vi "SCMP - Main Program v4.vi"() -> ()   [LabVIEW 2014]
doc: "Goodrich Exposure Range: .05microseconds to 798.9ms\n\nLow Gain (110e-/ADU)\nHigh Gain (6.5 e-/ADU)\n\nGA1280J Trigger Modes\n0 : Internally triggered; Internally timed\n1 : Externally triggered; Internally timed\n2 : Externally triggered; Externally timed\n3 : Externally gated; Internally timed\n\nFor list of camera commands\nsee Appendix A in the manual\n\n\nUse this template to build a standard state machine design pattern. Each state executes code and determines which state to transition to. Contrast this design pattern with the User Interface Event Handler pattern, in which code executes in response to user actions. Contrast this design pattern also with the Queued Message Handler pattern, in which each message handling code can queue zero or more new messages.\nNote: This template does not contain the most recent programming guidelines recommended by National Instruments. For a complete, project-based implementation of the Standard State Machine pattern, use the Create Project dialog box instead of this template."
uses:
  AISAS/Controls/Diffuser.ctl
  AISAS/Controls/Rotation.ctl
  PI/PI Control.ctl
  Controls/SCD - EDT - Emission Line Filter Wheel.ctl
  Controls/SCD - FITS Cluster.ctl
  AISAS/Mech/AISAS Mech.lvclass
  Controls/FITS Data type.ctl
  Controls/SCD - Calibration Optics Filter Wheel.ctl
  Controls/CoMP-S Controls/Polarization Optics Filter Wheel.ctl
  Controls/CoMP-S Controls/Emission Line Filter Wheel.ctl
  AISAS/Controls/focus.ctl
  Controls/peripherals.ctl
  Controls/Cameras select.ctl
  Controls/beaning.ctl
  Controls/Cookbook.ctl
  Controls/Cbk Data type.ctl
  Controls/Main Program States.ctl
  AISAS/Controls/motor.ctl
  AISAS/Mech/AISAS Mech.lvclass/AISAS Mech.ctl
  Camera/Andor Neo/Andor.lvclass
  Camera/Camera/Camera.lvclass
  Globals/Global - All Loop Stop.vi
  Globals/Global - pR netw comm.vi
  Controls/Globals.vi
  Controls/Global demo.vi
  c:/Users/mhutar/Documents/miro_lvproj/SCMP/Ancillary/Watlow EZ-ZONE/Public/Watbus.dll
  Ancillary/Watlow EZ-ZONE/Public/Watbus.dll
  <vilib>/Utility/error.llb/DialogType.ctl
panel:
  in  "Print scr1":bool
  in  "Comment":string="CoMP-S obs_prog_XXX"
  in  "Observer":string="Surname of the observer"
  out "Instrument":string
  out "Main Loop":bool
  out "Log Loop":bool
  out "Program":bool
  out "Version":string
  in  "AOI Width 2":i64=2560
  in  "AOI Height 2":i64=2160
  out "Latest Actions":string="\r"
  out "cbk name":string="automated_find_focus_656.cbk"
  out "Main Loop Error":errorcluster={"status"=TRUE, "code"=0, "source"=""}
  in  "Tab Control":T1(tab)
  in  "Auto scale":bool=TRUE
  in  "Live Preview":bool
  in  "Snap Images":bool
  out "Camera T Image Zoom":u16[][](graph)
  out "Histogram Graph 2":T2(graph)
  out "Timestamp 2":timestamp=timestamp(3507746192.5616717 s since 1904-01-01)
  out "Mean ADU 2":dbl=7788.0 format="%.1f"
  out "Sharpness 2":dbl format="%.2f"
  out "Camera FITS file path 2":path
  out "Camera R Image":u16[][](graph)
  in  "PI cam3 (mm)":T3 min=0.1 max=21.0 step=0.1 format="%.1f"
  in  "PI cam2 (mm)":T3 min=0.1 max=27.0 step=0.1 format="%.1f"
  in  "Calibration Optics":T4
  in  "Size":dbl format="%.2f"
  in  "Focus":T5 min=70.0 max=152.0 format="%.2f"
  in  "Andover Filter Wheel":T6
  in  "Calibration Wheel":T7
  in  "Binning":T8
  in  "Save Data to FITS?":bool
  out "Histogram Graph":T2(graph)
  in  "Exposure (s)":dbl=0.02 min=1e-05 max=10.0 step=0.001 format="%_3p"
  out "Timestamp":timestamp=timestamp(3507746192.5616717 s since 1904-01-01)
  in  "PI cam1 (mm)":T3 min=0.1 max=27.0 step=0.1 format="%.1f"
  out "Camera FITS file path":path
  in  "Emission Line Filters":T9
  in  "Set Filter Wheels":bool
  out "Mean ADU":dbl=7788.0 format="%.1f"
  out "Sharpness":dbl format="%.2f"
  in  "Diffuser":T10=enum."In Beam"
  in  "Rotation [deg]":T11 min=0.0 max=360.0 step=1.0 format="%.1f"
  in  "Move AISAS Mechanisms":bool
  in  "Motors":bool=TRUE
  out "Camera Image":u32[][](graph)
  out "Camera T Image":u16[][](graph)
  in  "Wavelength [nm]":dbl=557.0 min=0.0 step=0.01 format="%.2f"
  in  "Cameras":T12
  in  "preset cbk":u16(ring) caption="focus/filter/PIs/texp" items=["530.3nm (Fe XIV)", "587.6nm (He I D3)", "637.5nm (Fe X)", "656.3nm (H-Alpha)", "854.2nm (Ca I)", "1074.7nm (Fe XIII)", "1079.8nm (Fe XIII)", "1083.0nm (He I)"]
  in  "Setup Cor":bool
  in  "Looback disable":bool=TRUE caption="Disable Pointer Loopback\n  during Data aquisition"
  out "max Cookbook FPS":dbl=200.0 format="%#_3p"
  in  "Run Cookbook":bool
  in  "Save Data to FITS?":bool=TRUE
  out "Cookbook":T13=[{"Data Type"=enum."ACQUIRE DATA", "Arg 1"=0.0, "Arg 2"=0.0, "Arg 3"=path "", "Comments"=""}, {"Data Type"=enum."ACQUIRE DATA", "Arg 1"=0.0, "Arg 2"=0.0, "Arg 3"=path "", "Comments"=""}]
  out "FITS Path from Last Recipe Acquiring Data":path
  out "# of Recipes":i16
  out "Selected Cookbook":path
  out "Recipe Files":string[](array[string])
  in  "limit max Cookbook FPS to:":dbl=49.0 min=0.01 max=49.0 step=1.0 format="%_2f"
  out "Continually Read Log File":string="20160903-07:42:55 Live Preview Images\n20160903-07:44:38 Program Terminated\n20160903-07:45:16 Program Started\n20160903-07:45:18 Snap Single Image\n20160903-07:45:27 Live Preview Images\n20160903-07:46:17 Calibration & Filter wheel position:\t8\t5\n20160903-07:46:35 Live Preview Images\n20160903-07:50:39 Live Preview Images\n20160903-07:51:54 Camera Moved to Positon:-18.00\n20160903-07:51:55 Snap Single Image\n20160903-07:52:37 Loaded Cookbook\tfind_focus_656.cbk\n20160903-07:53:52 Run Cookbook\tfind_focus_656.cbk\n20160903-07:53:52 Recipe#0-exposure-20ms.rcp\n20160903-07:53:52 Recipe#1-fw-656.rcp\n20160903-07:53:54 Recipe#2-cal-open.rcp\n20160903-07:53:56 Recipe#3-move-absolute-neg19.rcp\n20160903-07:53:56 Recipe#4-take_656_focus_image.rcp\n20160903-07:54:02 Recipe#5-move-relative-neg0pt25.rcp\n20160903-07:55:56 Program Started\n20160903-07:56:02 Camera Moved to Positon:-18.00\n20160903-07:56:03 Snap Single Image\n20160903-07:56:35 Camera Moved to Positon:-19.00\n20160903-07:56:37 Snap Single Image\n20160903-07:56:58 Camera Moved to Positon:-20.00\n20160903-07:57:02 Snap Single Image\n20160903-07:57:20 Camera Moved to Positon:-21.00\n20160903-07:57:23 Snap Single Image\n20160903-07:57:36 Camera Moved to Positon:-22.00\n20160903-07:57:37 Snap Single Image\n20160903-07:57:53 Camera Moved to Positon:-25.00\n20160903-07:57:57 Snap Single Image\n20160903-07:58:13 Camera Moved to Positon:-30.00\n20160903-07:58:17 Snap Single Image\n20160903-07:58:43 Camera Moved to Positon:-18.00\n20160903-07:58:44 Snap Single Image\n20160903-07:58:58 Camera Moved to Positon:-17.00\n20160903-07:59:00 Snap Single Image\n20160903-08:00:39 Calibration & Filter wheel position:\t7\t6\n20160903-08:00:48 Snap Single Image\n20160903-08:01:42 Camera Moved to Positon:-65.00\n20160903-08:01:47 Snap Single Image\n20160903-08:02:07 Camera Moved to Positon:-70.00\n20160903-08:02:10 Snap Single Image\n20160903-08:02:51 Camera Moved to Positon:-75.00\n20160903-08:02:53 Snap Single Image\n20160903-08:03:25 Calibration & Filter wheel position:\t7\t7\n20160903-08:03:37 Snap Single Image\n20160903-08:03:55 Camera Moved to Positon:-76.00\n20160903-08:04:01 Snap Single Image\n20160903-08:04:13 Camera Moved to Positon:-77.00\n20160903-08:04:14 Snap Single Image\n20160903-08:04:24 Camera Moved to Positon:-78.00\n20160903-08:04:26 Snap Single Image\n20160903-08:04:38 Camera Moved to Positon:-79.00\n20160903-08:04:39 Snap Single Image\n20160903-08:04:50 Camera Moved to Positon:-83.00\n20160903-08:04:52 Snap Single Image\n20160903-08:05:10 Camera Moved to Positon:-73.00\n20160903-08:05:11 Snap Single Image\n20160903-08:05:22 Camera Moved to Positon:-71.00\n20160903-08:05:24 Snap Single Image\n20160903-08:05:34 Camera Moved to Positon:-69.00\n20160903-08:05:35 Snap Single Image\n20160903-08:05:47 Camera Moved to Positon:-67.00\n20160903-08:05:48 Snap Single Image\n20160903-08:06:13 Calibration & Filter wheel position:\t7\t8\n20160903-08:07:06 Snap Single Image\n20160903-08:07:17 Camera Moved to Positon:-69.00\n20160903-08:07:18 Snap Single Image\n20160903-08:07:28 Camera Moved to Positon:-71.00\n20160903-08:07:30 Snap Single Image\n20160903-08:07:40 Camera Moved to Positon:-73.00\n20160903-08:07:43 Snap Single Image\n20160903-08:07:53 Camera Moved to Positon:-75.00\n20160903-08:07:55 Snap Single Image\n20160903-08:08:04 Camera Moved to Positon:-77.00\n20160903-08:08:06 Snap Single Image\n20160903-08:08:17 Camera Moved to Positon:-79.00\n20160903-08:08:28 Snap Single Image\n20160903-08:08:43 Camera Moved to Positon:-81.00\n20160903-08:08:46 Snap Single Image\n20160903-08:09:05 Calibration & Filter wheel position:\t7\t9\n20160903-08:09:48 Camera Moved to Positon:-100.00\n20160903-08:09:50 Snap Single Image\n20160903-08:10:09 Snap Single Image\n20160903-08:10:26 Camera Moved to Positon:-100.00\n20160903-08:10:35 Camera Moved to Positon:-100.00\n20160903-08:10:37 Snap Single Image\n20160903-08:10:54 Camera Moved to Positon:-100.00\n20160903-08:10:59 Program Terminated\n20160903-08:12:25 Program Started\n20160903-08:12:33 Camera Moved to Positon:-100.00\n20160903-08:12:38 Program Terminated\n20160903-08:13:25 Program Started\n20160903-08:13:30 Camera Moved to Positon:-100.00\n20160903-08:13:37 Program Terminated\n20160903-08:14:12 Program Started\n20160903-08:14:19 Camera Moved to Positon:-100.00\n20160903-08:14:22 Snap Single Image\n20160903-08:14:37 Calibration & Filter wheel position:\t7\t9\n20160903-08:14:45 Snap Single Image\n20160903-08:14:56 Camera Moved to Positon:-105.00\n20160903-08:14:57 Snap Single Image\n20160903-08:15:10 Camera Moved to Positon:-110.00\n20160903-08:15:11 Snap Single Image\n20160903-08:15:23 Camera Moved to Positon:-115.00\n20160903-08:15:27 Snap Single Image\n20160903-08:15:39 Camera Moved to Positon:-120.00\n20160903-08:15:40 Snap Single Image\n20160903-08:15:59 Snap Single Image\n20160903-08:16:10 Camera Moved to Positon:-115.00\n20160903-08:16:11 Snap Single Image\n20160903-08:16:21 Camera Moved to Positon:-110.00\n20160903-08:16:22 Snap Single Image\n20160903-08:16:33 Camera Moved to Positon:-105.00\n20160903-08:16:36 Snap Single Image\n20160903-08:16:49 Camera Moved to Positon:-100.00\n20160903-08:16:51 Snap Single Image\n20160903-08:17:03 Camera Moved to Positon:-95.00\n20160903-08:17:05 Snap Single Image\n20160903-08:17:16 Camera Moved to Positon:-90.00\n20160903-08:17:18 Snap Single Image\n20160903-08:17:46 Camera Moved to Positon:-85.00\n20160903-08:17:49 Snap Single Image\n20160903-08:18:00 Camera Moved to Positon:-80.00\n20160903-08:18:02 Snap Single Image\n20160903-08:18:40 Calibration & Filter wheel position:\t7\t4\n20160903-08:18:59 Camera Moved to Positon:-20.00\n20160903-08:19:11 Snap Single Image\n20160903-08:19:23 Camera Moved to Positon:-18.00\n20160903-08:19:25 Snap Single Image\n20160903-08:19:38 Camera Moved to Positon:-22.00\n20160903-08:19:39 Snap Single Image\n20160903-08:19:51 Camera Moved to Positon:-24.00\n20160903-08:19:52 Snap Single Image\n20160903-08:20:04 Calibration & Filter wheel position:\t7\t3\n20160903-08:20:11 Snap Single Image\n20160903-08:20:22 Camera Moved to Positon:-18.00\n20160903-08:20:24 Snap Single Image\n20160903-08:20:39 Camera Moved to Positon:-16.00\n20160903-08:20:40 Snap Single Image\n20160903-08:20:53 Camera Moved to Positon:-14.00\n20160903-08:20:56 Snap Single Image\n20160903-08:21:06 Camera Moved to Positon:-12.00\n20160903-08:21:07 Snap Single Image\n20160903-08:21:16 Camera Moved to Positon:-10.00\n20160903-08:21:24 Snap Single Image\n20160903-08:21:34 Camera Moved to Positon: -8.00\n20160903-08:21:36 Snap Single Image\n20160903-08:22:12 Camera Moved to Positon: -6.00\n20160903-08:22:21 Snap Single Image\n20160903-08:23:09 Calibration & Filter wheel position:\t7\t1\n20160903-08:23:17 Snap Single Image\n20160903-08:23:27 Camera Moved to Positon: -4.00\n20160903-08:23:29 Snap Single Image\n20160903-08:23:37 Camera Moved to Positon: -2.00\n20160903-08:23:38 Snap Single Image\n20160903-08:23:47 Camera Moved to Positon:  0.00\n20160903-08:23:50 Snap Single Image\n20160903-08:26:00 Camera Moved to Positon:-18.00\n20160903-08:26:44 Program Started\n20160903-08:26:59 Camera Moved to Positon:-18.00\n20160903-08:27:05 Loaded Cookbook\tfind_focus_656.cbk\n20160903-08:27:12 Run Cookbook\tfind_focus_656.cbk\n20160903-08:27:12 Recipe#0-exposure-20ms.rcp\n20160903-08:27:12 Recipe#1-fw-656.rcp\n20160903-08:27:14 Recipe#2-cal-open.rcp\n20160903-08:27:16 Recipe#3-take_656_focus_image.rcp\n20160903-08:29:11 Camera Moved to Positon:-19.00\n20160903-08:29:17 Run Cookbook\tfind_focus_656.cbk\n20160903-08:29:17 Recipe#0-exposure-20ms.rcp\n20160903-08:29:17 Recipe#1-fw-656.rcp\n20160903-08:29:19 Recipe#2-cal-open.rcp\n20160903-08:29:21 Recipe#3-take_656_focus_image.rcp\n20160903-08:29:59 Camera Moved to Positon:-20.00\n20160903-08:30:03 Run Cookbook\tfind_focus_656.cbk\n20160903-08:30:03 Recipe#0-exposure-20ms.rcp\n20160903-08:30:03 Recipe#1-fw-656.rcp\n20160903-08:30:05 Recipe#2-cal-open.rcp\n20160903-08:30:07 Recipe#3-take_656_focus_image.rcp\n20160903-08:30:28 Camera Moved to Positon:-21.00\n20160903-08:30:32 Run Cookbook\tfind_focus_656.cbk\n20160903-08:30:32 Recipe#0-exposure-20ms.rcp\n20160903-08:30:32 Recipe#1-fw-656.rcp\n20160903-08:30:34 Recipe#2-cal-open.rcp\n20160903-08:30:36 Recipe#3-take_656_focus_image.rcp\n20160903-08:31:03 Camera Moved to Positon:-22.00\n20160903-08:31:06 Run Cookbook\tfind_focus_656.cbk\n20160903-08:31:06 Recipe#0-exposure-20ms.rcp\n20160903-08:31:06 Recipe#1-fw-656.rcp\n20160903-08:31:08 Recipe#2-cal-open.rcp\n20160903-08:31:10 Recipe#3-take_656_focus_image.rcp\n20160903-08:31:33 Camera Moved to Positon:-23.00\n20160903-08:31:38 Run Cookbook\tfind_focus_656.cbk\n20160903-08:31:38 Recipe#0-exposure-20ms.rcp\n20160903-08:31:38 Recipe#1-fw-656.rcp\n20160903-08:31:40 Recipe#2-cal-open.rcp\n20160903-08:31:42 Recipe#3-take_656_focus_image.rcp\n20160903-08:32:05 Camera Moved to Positon:-24.00\n20160903-08:32:08 Run Cookbook\tfind_focus_656.cbk\n20160903-08:32:08 Recipe#0-exposure-20ms.rcp\n20160903-08:32:08 Recipe#1-fw-656.rcp\n20160903-08:32:10 Recipe#2-cal-open.rcp\n20160903-08:32:12 Recipe#3-take_656_focus_image.rcp\n20160903-08:32:35 Camera Moved to Positon:-25.00\n20160903-08:32:40 Run Cookbook\tfind_focus_656.cbk\n20160903-08:32:40 Recipe#0-exposure-20ms.rcp\n20160903-08:32:40 Recipe#1-fw-656.rcp\n20160903-08:32:42 Recipe#2-cal-open.rcp\n20160903-08:32:44 Recipe#3-take_656_focus_image.rcp\n20160903-08:33:03 Camera Moved to Positon:-26.00\n20160903-08:33:07 Run Cookbook\tfind_focus_656.cbk\n20160903-08:33:07 Recipe#0-exposure-20ms.rcp\n20160903-08:33:07 Recipe#1-fw-656.rcp\n20160903-08:33:09 Recipe#2-cal-open.rcp\n20160903-08:33:11 Recipe#3-take_656_focus_image.rcp\n20160903-08:33:32 Camera Moved to Positon:-27.00\n20160903-08:33:34 Run Cookbook\tfind_focus_656.cbk\n20160903-08:33:34 Recipe#0-exposure-20ms.rcp\n20160903-08:33:34 Recipe#1-fw-656.rcp\n20160903-08:33:36 Recipe#2-cal-open.rcp\n20160903-08:33:38 Recipe#3-take_656_focus_image.rcp\n20160903-08:34:01 Camera Moved to Positon:-28.00\n20160903-08:34:05 Run Cookbook\tfind_focus_656.cbk\n20160903-08:34:05 Recipe#0-exposure-20ms.rcp\n20160903-08:34:05 Recipe#1-fw-656.rcp\n20160903-08:34:07 Recipe#2-cal-open.rcp\n20160903-08:34:09 Recipe#3-take_656_focus_image.rcp\n20160903-08:36:44 Camera Moved to Positon:-85.00\n20160903-08:36:51 Loaded Cookbook\tfind_focus_1083.cbk\n20160903-08:37:11 Loaded Cookbook\tfind_focus_1083.cbk\n20160903-08:37:20 Run Cookbook\tfind_focus_1083.cbk\n20160903-08:37:20 Recipe#0-exposure-120ms.rcp\n20160903-08:37:20 Recipe#1-fw-1083.rcp\n20160903-08:37:22 Recipe#2-cal-open.rcp\n20160903-08:37:23 Recipe#3-take_1083_focus_image.rcp\n20160903-08:38:05 Camera Moved to Positon:-86.00\n20160903-08:38:11 Run Cookbook\tfind_focus_1083.cbk\n20160903-08:38:11 Recipe#0-exposure-120ms.rcp\n20160903-08:38:11 Recipe#1-fw-1083.rcp\n20160903-08:38:13 Recipe#2-cal-open.rcp\n20160903-08:38:15 Recipe#3-take_1083_focus_image.rcp\n20160903-08:38:39 Camera Moved to Positon:-87.00\n20160903-08:38:43 Run Cookbook\tfind_focus_1083.cbk\n20160903-08:38:43 Recipe#0-exposure-120ms.rcp\n20160903-08:38:43 Recipe#1-fw-1083.rcp\n20160903-08:38:45 Recipe#2-cal-open.rcp\n20160903-08:38:47 Recipe#3-take_1083_focus_image.rcp\n20160903-08:39:05 Camera Moved to Positon:-88.00\n20160903-08:39:09 Run Cookbook\tfind_focus_1083.cbk\n20160903-08:39:10 Recipe#0-exposure-120ms.rcp\n20160903-08:39:10 Recipe#1-fw-1083.rcp\n20160903-08:39:12 Recipe#2-cal-open.rcp\n20160903-08:39:13 Recipe#3-take_1083_focus_image.rcp\n20160903-08:43:45 Snap Single Image\n20160903-08:43:56 Run Cookbook\tfind_focus_1083.cbk\n20160903-08:43:56 Recipe#0-exposure-120ms.rcp\n20160903-08:43:56 Recipe#1-fw-1083.rcp\n20160903-08:43:58 Recipe#2-cal-open.rcp\n20160903-08:44:00 Recipe#3-take_1083_focus_image.rcp\n20160903-08:44:24 Camera Moved to Positon:-90.00\n20160903-08:44:32 Camera Moved to Positon:-89.00\n20160903-08:44:36 Run Cookbook\tfind_focus_1083.cbk\n20160903-08:44:36 Recipe#0-exposure-120ms.rcp\n20160903-08:44:36 Recipe#1-fw-1083.rcp\n20160903-08:44:38 Recipe#2-cal-open.rcp\n20160903-08:44:40 Recipe#3-take_1083_focus_image.rcp\n20160903-08:45:03 Camera Moved to Positon:-90.00\n20160903-08:45:11 Run Cookbook\tfind_focus_1083.cbk\n20160903-08:45:12 Recipe#0-exposure-120ms.rcp\n20160903-08:45:12 Recipe#1-fw-1083.rcp\n20160903-08:45:14 Recipe#2-cal-open.rcp\n20160903-08:45:15 Recipe#3-take_1083_focus_image.rcp\n20160903-08:45:38 Camera Moved to Positon:-91.00\n20160903-08:45:41 Run Cookbook\tfind_focus_1083.cbk\n20160903-08:45:41 Recipe#0-exposure-120ms.rcp\n20160903-08:45:42 Recipe#1-fw-1083.rcp\n20160903-08:45:43 Recipe#2-cal-open.rcp\n20160903-08:45:45 Recipe#3-take_1083_focus_image.rcp\n20160903-08:46:07 Camera Moved to Positon:-92.00\n20160903-08:46:12 Run Cookbook\tfind_focus_1083.cbk\n20160903-08:46:12 Recipe#0-exposure-120ms.rcp\n20160903-08:46:12 Recipe#1-fw-1083.rcp\n20160903-08:46:14 Recipe#2-cal-open.rcp\n20160903-08:46:16 Recipe#3-take_1083_focus_image.rcp\n20160903-08:46:53 Camera Moved to Positon:-93.00\n20160903-08:46:56 Run Cookbook\tfind_focus_1083.cbk\n20160903-08:46:56 Recipe#0-exposure-120ms.rcp\n20160903-08:46:56 Recipe#1-fw-1083.rcp\n20160903-08:46:58 Recipe#2-cal-open.rcp\n20160903-08:47:00 Recipe#3-take_1083_focus_image.rcp\n20160903-08:48:13 Calibration & Filter wheel position:\t7\t3\n20160903-08:51:11 Camera Moved to Positon:-10.00\n20160903-08:51:19 Camera Moved to Positon: -5.00\n20160903-08:51:20 Live Preview Images\n20160903-08:51:43 Loaded Cookbook\tfind_focus_589.cbk\n20160903-08:52:08 Loaded Cookbook\tfocus-656.cbk\n20160903-08:52:09 Run Cookbook\tfocus-656.cbk\n20160903-08:52:09 Recipe#0-fw-656.rcp\n20160903-08:52:11 Recipe#1-cal-clear.rcp\n20160903-08:52:13 Recipe#2-exposure-200ms.rcp\n20160903-08:52:13 Recipe#3-focus-656.rcp\n20160903-08:52:24 Program Started\n20160903-08:52:33 Loaded Cookbook\tfocus-656.cbk\n20160903-08:52:40 Camera Moved to Positon: -5.00\n20160903-08:52:46 Loaded Cookbook\tfind_focus_589.cbk\n20160903-08:52:48 Run Cookbook\tfind_focus_589.cbk\n20160903-08:52:48 Recipe#0-exposure-20ms.rcp\n20160903-08:52:48 Recipe#1-fw-589.rcp\n20160903-08:52:50 Recipe#2-cal-open.rcp\n20160903-08:52:52 Recipe#3-take_589_focus_image.rcp\n20160903-08:54:55 Run Cookbook\tfind_focus_589.cbk\n20160903-08:54:55 Recipe#0-exposure-20ms.rcp\n20160903-08:54:56 Recipe#1-fw-589.rcp\n20160903-08:54:57 Recipe#2-cal-open.rcp\n20160903-08:54:59 Recipe#3-take_589_focus_image.rcp\n20160903-08:55:19 Live Preview Images\n20160903-08:56:01 Camera Moved to Positon: -6.00\n20160903-08:56:04 Run Cookbook\tfind_focus_589.cbk\n20160903-08:56:04 Recipe#0-exposure-20ms.rcp\n20160903-08:56:04 Recipe#1-fw-589.rcp\n20160903-08:56:06 Recipe#2-cal-open.rcp\n20160903-08:56:08 Recipe#3-take_589_focus_image.rcp\n20160903-08:56:40 Camera Moved to Positon: -7.00\n20160903-08:58:30 Run Cookbook\tfind_focus_589.cbk\n20160903-08:58:30 Recipe#0-exposure-20ms.rcp\n20160903-08:58:30 Recipe#1-fw-589.rcp\n20160903-08:58:32 Recipe#2-cal-open.rcp\n20160903-08:58:34 Recipe#3-take_589_focus_image.rcp\n20160903-08:59:22 Camera Moved to Positon: -8.00\n20160903-09:14:18 Program Terminated\n20160903-09:40:55 Program Started\n20160903-09:44:03 Loaded Cookbook\tautomated_find_focus_656.cbk\n20160903-09:44:43 Loaded Cookbook\tautomated_find_focus_656.cbk\n20160903-09:44:57 Run Cookbook\tautomated_find_focus_656.cbk\n20160903-09:44:57 Recipe#0-exposure-20ms.rcp\n20160903-09:44:57 Recipe#1-fw-656.rcp\n20160903-09:44:59 Recipe#2-cal-open.rcp\n20160903-09:45:01 Recipe#3-move-absolute-neg15.rcp\n20160903-09:45:02 Recipe#4-take_656_focus_image.rcp\n20160903-09:45:16 Recipe#5-move-relative-neg0pt25.rcp\n20160903-09:45:17 Recipe#6-take_656_focus_image.rcp\n20160903-09:45:31 Recipe#7-move-relative-neg0pt25.rcp\n20160903-09:45:32 Recipe#8-take_656_focus_image.rcp\n20160903-09:45:46 Recipe#9-move-relative-neg0pt25.rcp\n20160903-09:45:47 Recipe#10-take_656_focus_image.rcp\n20160903-09:46:01 Recipe#11-move-relative-neg0pt25.rcp\n20160903-09:46:02 Recipe#12-take_656_focus_image.rcp\n20160903-09:46:17 Recipe#13-move-relative-neg0pt25.rcp\n20160903-09:46:18 Recipe#14-take_656_focus_image.rcp\n20160903-09:46:32 Recipe#15-move-relative-neg0pt25.rcp\n20160903-09:46:33 Recipe#16-take_656_focus_image.rcp\n20160903-09:46:47 Recipe#17-move-relative-neg0pt25.rcp\n20160903-09:46:48 Recipe#18-take_656_focus_image.rcp\n20160903-09:47:02 Recipe#19-move-relative-neg0pt25.rcp\n20160903-09:47:03 Recipe#20-take_656_focus_image.rcp\n20160903-09:47:17 Recipe#21-move-relative-neg0pt25.rcp\n20160903-09:47:17 Recipe#22-take_656_focus_image.rcp\n20160903-09:47:32 Recipe#23-move-relative-neg0pt25.rcp\n20160903-09:47:32 Recipe#24-take_656_focus_image.rcp\n20160903-09:47:46 Recipe#25-move-relative-neg0pt25.rcp\n20160903-09:47:47 Recipe#26-take_656_focus_image.rcp\n20160903-09:48:02 Recipe#27-move-relative-neg0pt25.rcp\n20160903-09:48:03 Recipe#28-take_656_focus_image.rcp\n20160903-09:48:17 Recipe#29-move-relative-neg0pt25.rcp\n20160903-09:48:17 Recipe#30-take_656_focus_image.rcp\n20160903-09:48:32 Recipe#31-move-relative-neg0pt25.rcp\n20160903-09:48:33 Recipe#32-take_656_focus_image.rcp\n20160903-09:48:49 Recipe#33-move-relative-neg0pt25.rcp\n20160903-09:48:49 Recipe#34-take_656_focus_image.rcp\n20160903-09:49:05 Recipe#35-move-relative-neg0pt25.rcp\n20160903-09:49:06 Recipe#36-take_656_focus_image.rcp\n20160903-09:49:23 Recipe#37-move-relative-neg0pt25.rcp\n20160903-09:49:24 Recipe#38-take_656_focus_image.rcp\n20160903-09:49:41 Recipe#39-move-relative-neg0pt25.rcp\n20160903-09:49:42 Recipe#40-take_656_focus_image.rcp\n20160903-09:50:01 Recipe#41-move-relative-neg0pt25.rcp\n20160903-09:50:01 Recipe#42-take_656_focus_image.rcp\n20160903-09:50:20 Recipe#43-move-relative-neg0pt25.rcp\n20160903-09:50:21 Recipe#44-take_656_focus_image.rcp\n20160903-09:54:36 Loaded Cookbook\tautomated_find_focus_656.cbk\n20160903-09:54:47 Loaded Cookbook\tautomated_find_focus_656.cbk\n20160903-09:55:40 Loaded Cookbook\tautomated_find_focus_656.cbk\n20160903-09:55:54 Run Cookbook\tautomated_find_focus_656.cbk\n20160903-09:55:54 Recipe#0-exposure-40ms.rcp\n20160903-09:55:54 Recipe#1-fw-656.rcp\n20160903-09:55:56 Recipe#2-cal-open.rcp\n20160903-09:55:58 Recipe#3-move-absolute-neg15.rcp\n20160903-09:55:59 Recipe#4-take_656_focus_image.rcp\n20160903-09:56:06 Recipe#5-move-relative-neg0pt5.rcp\n20160903-09:56:07 Recipe#6-take_656_focus_image.rcp\n20160903-09:56:14 Recipe#7-move-relative-neg0pt5.rcp\n20160903-09:56:15 Recipe#8-take_656_focus_image.rcp\n20160903-09:56:22 Recipe#9-move-relative-neg0pt5.rcp\n20160903-09:56:22 Recipe#10-take_656_focus_image.rcp\n20160903-09:56:29 Recipe#11-move-relative-neg0pt5.rcp\n20160903-09:56:30 Recipe#12-take_656_focus_image.rcp\n20160903-09:56:37 Recipe#13-move-relative-neg0pt5.rcp\n20160903-09:56:38 Recipe#14-take_656_focus_image.rcp\n20160903-09:56:45 Recipe#15-move-relative-neg0pt5.rcp\n20160903-09:56:45 Recipe#16-take_656_focus_image.rcp\n20160903-09:56:52 Recipe#17-move-relative-neg0pt5.rcp\n20160903-09:56:53 Recipe#18-take_656_focus_image.rcp\n20160903-09:57:00 Recipe#19-move-relative-neg0pt5.rcp\n20160903-09:57:01 Recipe#20-take_656_focus_image.rcp\n20160903-09:57:08 Recipe#21-move-relative-neg0pt5.rcp\n20160903-09:57:09 Recipe#22-take_656_focus_image.rcp\n20160903-09:57:16 Recipe#23-move-relative-neg0pt5.rcp\n20160903-09:57:16 Recipe#24-take_656_focus_image.rcp\n20160903-09:57:23 Recipe#25-move-relative-neg0pt5.rcp\n20160903-09:57:24 Recipe#26-take_656_focus_image.rcp\n20160903-09:57:31 Recipe#27-move-relative-neg0pt5.rcp\n20160903-09:57:32 Recipe#28-take_656_focus_image.rcp\n20160903-09:57:39 Recipe#29-move-relative-neg0pt5.rcp\n20160903-09:57:40 Recipe#30-take_656_focus_image.rcp\n20160903-09:57:47 Recipe#31-move-relative-neg0pt5.rcp\n20160903-09:57:48 Recipe#32-take_656_focus_image.rcp\n20160903-09:57:55 Recipe#33-move-relative-neg0pt5.rcp\n20160903-09:57:56 Recipe#34-take_656_focus_image.rcp\n20160903-09:58:03 Recipe#35-move-relative-neg0pt5.rcp\n20160903-09:58:03 Recipe#36-take_656_focus_image.rcp\n20160903-09:58:10 Recipe#37-move-relative-neg0pt5.rcp\n20160903-09:58:11 Recipe#38-take_656_focus_image.rcp\n20160903-09:58:18 Recipe#39-move-relative-neg0pt5.rcp\n20160903-09:58:19 Recipe#40-take_656_focus_image.rcp\n20160903-09:58:26 Recipe#41-move-relative-neg0pt5.rcp\n20160903-09:58:27 Recipe#42-take_656_focus_image.rcp\n20160903-09:58:34 Recipe#43-move-relative-neg0pt5.rcp\n20160903-09:58:35 Recipe#44-take_656_focus_image.rcp\n20160903-10:46:33 Program Terminated\n20160903-12:25:32 Program Started\n20160903-12:26:22 Program Terminated\n20160903-12:45:45 Program Started\n20160903-12:45:56 Program Terminated\n20160903-12:49:12 Program Started\n20160903-12:49:15 Loaded Cookbook\tautomated_find_focus_656.cbk\n20160903-12:49:24 Run Cookbook\tautomated_find_focus_656.cbk\n20160903-12:49:25 Recipe#0-exposure-40ms.rcp\n20160903-12:49:25 Recipe#1-fw-656.rcp\n20160903-12:49:26 Recipe#2-cal-open.rcp\n20160903-12:49:28 Recipe#3-move-absolute-neg15.rcp\n20160903-12:49:29 Recipe#4-take_656_focus_image.rcp\n20160903-12:49:32 Recipe#5-move-relative-neg0pt5.rcp\n20160903-12:49:33 Recipe#6-take_656_focus_image.rcp\n20160903-12:49:36 Recipe#7-move-relative-neg0pt5.rcp\n20160903-12:49:36 Recipe#8-take_656_focus_image.rcp\n20160903-12:49:39 Recipe#9-move-relative-neg0pt5.rcp\n20160903-12:49:40 Recipe#10-take_656_focus_image.rcp\n20160903-12:49:43 Recipe#11-move-relative-neg0pt5.rcp\n20160903-12:49:43 Recipe#12-take_656_focus_image.rcp\n20160903-12:49:46 Recipe#13-move-relative-neg0pt5.rcp\n20160903-12:49:47 Recipe#14-take_656_focus_image.rcp\n20160903-12:49:49 Recipe#15-move-relative-neg0pt5.rcp\n20160903-12:49:50 Recipe#16-take_656_focus_image.rcp\n20160903-12:49:53 Recipe#17-move-relative-neg0pt5.rcp\n20160903-12:49:53 Recipe#18-take_656_focus_image.rcp\n20160903-12:49:56 Recipe#19-move-relative-neg0pt5.rcp\n20160903-12:49:57 Recipe#20-take_656_focus_image.rcp\n20160903-12:49:59 Recipe#21-move-relative-neg0pt5.rcp\n20160903-12:50:00 Recipe#22-take_656_focus_image.rcp\n20160903-12:50:03 Recipe#23-move-relative-neg0pt5.rcp\n20160903-12:50:04 Recipe#24-take_656_focus_image.rcp\n20160903-12:50:06 Recipe#25-move-relative-neg0pt5.rcp\n20160903-12:50:07 Recipe#26-take_656_focus_image.rcp\n20160903-12:50:10 Recipe#27-move-relative-neg0pt5.rcp\n20160903-12:50:10 Recipe#28-take_656_focus_image.rcp\n20160903-12:50:13 Recipe#29-move-relative-neg0pt5.rcp\n20160903-12:50:14 Recipe#30-take_656_focus_image.rcp\n20160903-12:50:16 Recipe#31-move-relative-neg0pt5.rcp\n20160903-12:50:17 Recipe#32-take_656_focus_image.rcp\n20160903-12:50:20 Recipe#33-move-relative-neg0pt5.rcp\n20160903-12:50:20 Recipe#34-take_656_focus_image.rcp\n20160903-12:50:23 Recipe#35-move-relative-neg0pt5.rcp\n20160903-12:50:24 Recipe#36-take_656_focus_image.rcp\n20160903-12:50:26 Recipe#37-move-relative-neg0pt5.rcp\n20160903-12:50:27 Recipe#38-take_656_focus_image.rcp\n20160903-12:50:30 Recipe#39-move-relative-neg0pt5.rcp\n20160903-12:50:31 Recipe#40-take_656_focus_image.rcp\n20160903-12:50:33 Recipe#41-move-relative-neg0pt5.rcp\n20160903-12:50:34 Recipe#42-take_656_focus_image.rcp\n20160903-12:50:37 Recipe#43-move-relative-neg0pt5.rcp\n20160903-12:50:37 Recipe#44-take_656_focus_image.rcp\n20160903-13:54:17 Program Terminated\n20160903-14:07:18 Program Started\n20160903-14:08:12 Program Terminated\n20160903-14:20:46 Program Started\n20160903-14:22:56 Program Terminated\n20160903-14:23:20 Program Started\n20160903-14:25:03 Program Terminated\n20160903-14:31:16 Program Started\n20160903-14:32:59 Program Terminated\n20160903-14:33:26 Program Started\n20160903-14:35:01 Program Terminated\n20160903-14:36:43 Program Started\n20160903-14:38:01 Program Terminated\n20160903-14:39:22 Program Started\n20160903-14:39:47 Program Terminated\n20160903-14:40:22 Program Started\n20160903-14:41:59 Program Terminated\n20160903-15:07:40 Program Started\n20160903-15:10:18 Program Terminated\n20160903-15:19:59 Program Started\n20160903-15:20:17 Program Terminated\n20160903-15:20:43 Program Started\n20160903-15:20:43 Program Terminated\n20160903-15:21:33 Program Started\n20160903-15:22:45 Program Terminated\n20160903-15:24:43 Program Started\n20160903-15:26:40 Program Terminated\n20160903-15:29:07 Program Started\n20160903-15:29:52 Loaded Cookbook\tautomated_find_focus_656.cbk\n20160903-15:30:08 Loaded Cookbook\tautomated_find_focus_656.cbk\n"
  out "min Cookbook Exposure [s]":dbl format="%#_3p"
  out "Today's SCMP Log File":path
  out "Cookbook Comments":string
  in  "Mod/Seq":bool
  in  "Load Cookbook":bool
  in  "Pointer IP":string="127.0.0.1"
  out "Network\nconnected":bool
  out "Pointer ON":bool
  in  "Enable Data Logging":bool=TRUE
  out "Today's SCMP Eng  File":path
  out "Air around \nprefilter wheel [C]":sgl(graph)
  out "Lyot Filter Temp [C]":dbl(graph)
  out "Air around Camera [C]":sgl(graph)
  out "Air around Lyot Filter [C]":dbl(graph)
  out "Eng Data Error":errorcluster={"status"=TRUE, "code"=0, "source"=""}
  out "Camera 1 Temp [C}":dbl(graph)=-21.03
  out "Camera 2 Temp [C}":dbl(graph)=-21.03
  in  "AISAS verification":bool=TRUE
  out "Processing":bool
  out "Calib image":u32[][](graph)
  in  "Run Dark":bool
  in  "Dark/Flat":bool
  in  "Dark/Flat2":bool
  out "FITS Header":T15={"Wavelength (nm)"=530.15, "Exposure (s)"=0.05, "Tuning Delay (ms)"=1000.0, "Beam Type (-1/1)"=1.0, "Tuning Voltages"=[1.111, 2.222, 3.333, 4.444], "Observer"="observer", "Light Shapping Diffuser"=enum."In Beam", "Comment"="", "Data Type"=enum."HOLE", "Mod Cycles"=0, "SCD Calibration Optics"=enum."1 - Polarizer @0, I+Q", "SCD Emission Line Filter"=enum."1-557.6nm", "Cookbook"="", "COMP-S Calibration Wheel"=enum."Dark", "COMP-S Andover Filter Wheel"=enum."530.3nm/HWB 0.34nm (Fe XIV)", "FOV Rotation (deg)"=66.0, "Objective Lens Position (mm)"=0.0, "Occulter size"=0.0, "Time End"=timestamp(3382374145.421875 s since 1904-01-01), "Acc Exposure (s)"=0.0, "Time Stamp Array"=[], "Camera Serial Number"=[], "Camera Temp"=[], "Camera PI (mm)"=[], "Time Start"=timestamp(3382374145.421875 s since 1904-01-01), "Peripherals"={"ILX controler"=FALSE, "Zone temperatures"=FALSE, "Andor"=FALSE, "Andor 2"=FALSE, "PI Stages"=FALSE, "AISAS mechanisms"=FALSE, "AISAS Mech.lvclass"=refnum, "Zone temp ref"=variant, "FWs"=FALSE}, "FITS paths"=[], "Cameras"=enum."Andor", "load preset cbk"=FALSE, "periodic check count"=0, "COMP-S Calibration Wheel 2"=enum."Dark", "Calib"=enum."Dark", "Abso Aperture"=66.0, "Nominal Aperture"=66.0, "Pointer IP"="127.0.0.1"} {"Nominal Aperture" format="%.1f"; "Abso Aperture" format="%.1f"; "Camera PI (mm)" format="%_3g"; "Acc Exposure (s)" format="%^.3g"; "Occulter size" format="%.2f"; "Objective Lens Position (mm)" min=70.0 max=152.0 format="%.2f"; "FOV Rotation (deg)" format="%.1f"; "Exposure (s)" format="%^.3g"; "Wavelength (nm)" format="%_6g"}
  in  "Andor Adv Settings":bool
  in  "scmp nohyde":bool
  in  "Stop":bool=TRUE
  # "Camera Settings"
  # "Filter Wheels"
  # "Coronograph+Instrument Setup"
  # "AISAS mechanisms"
  # "Occulter"
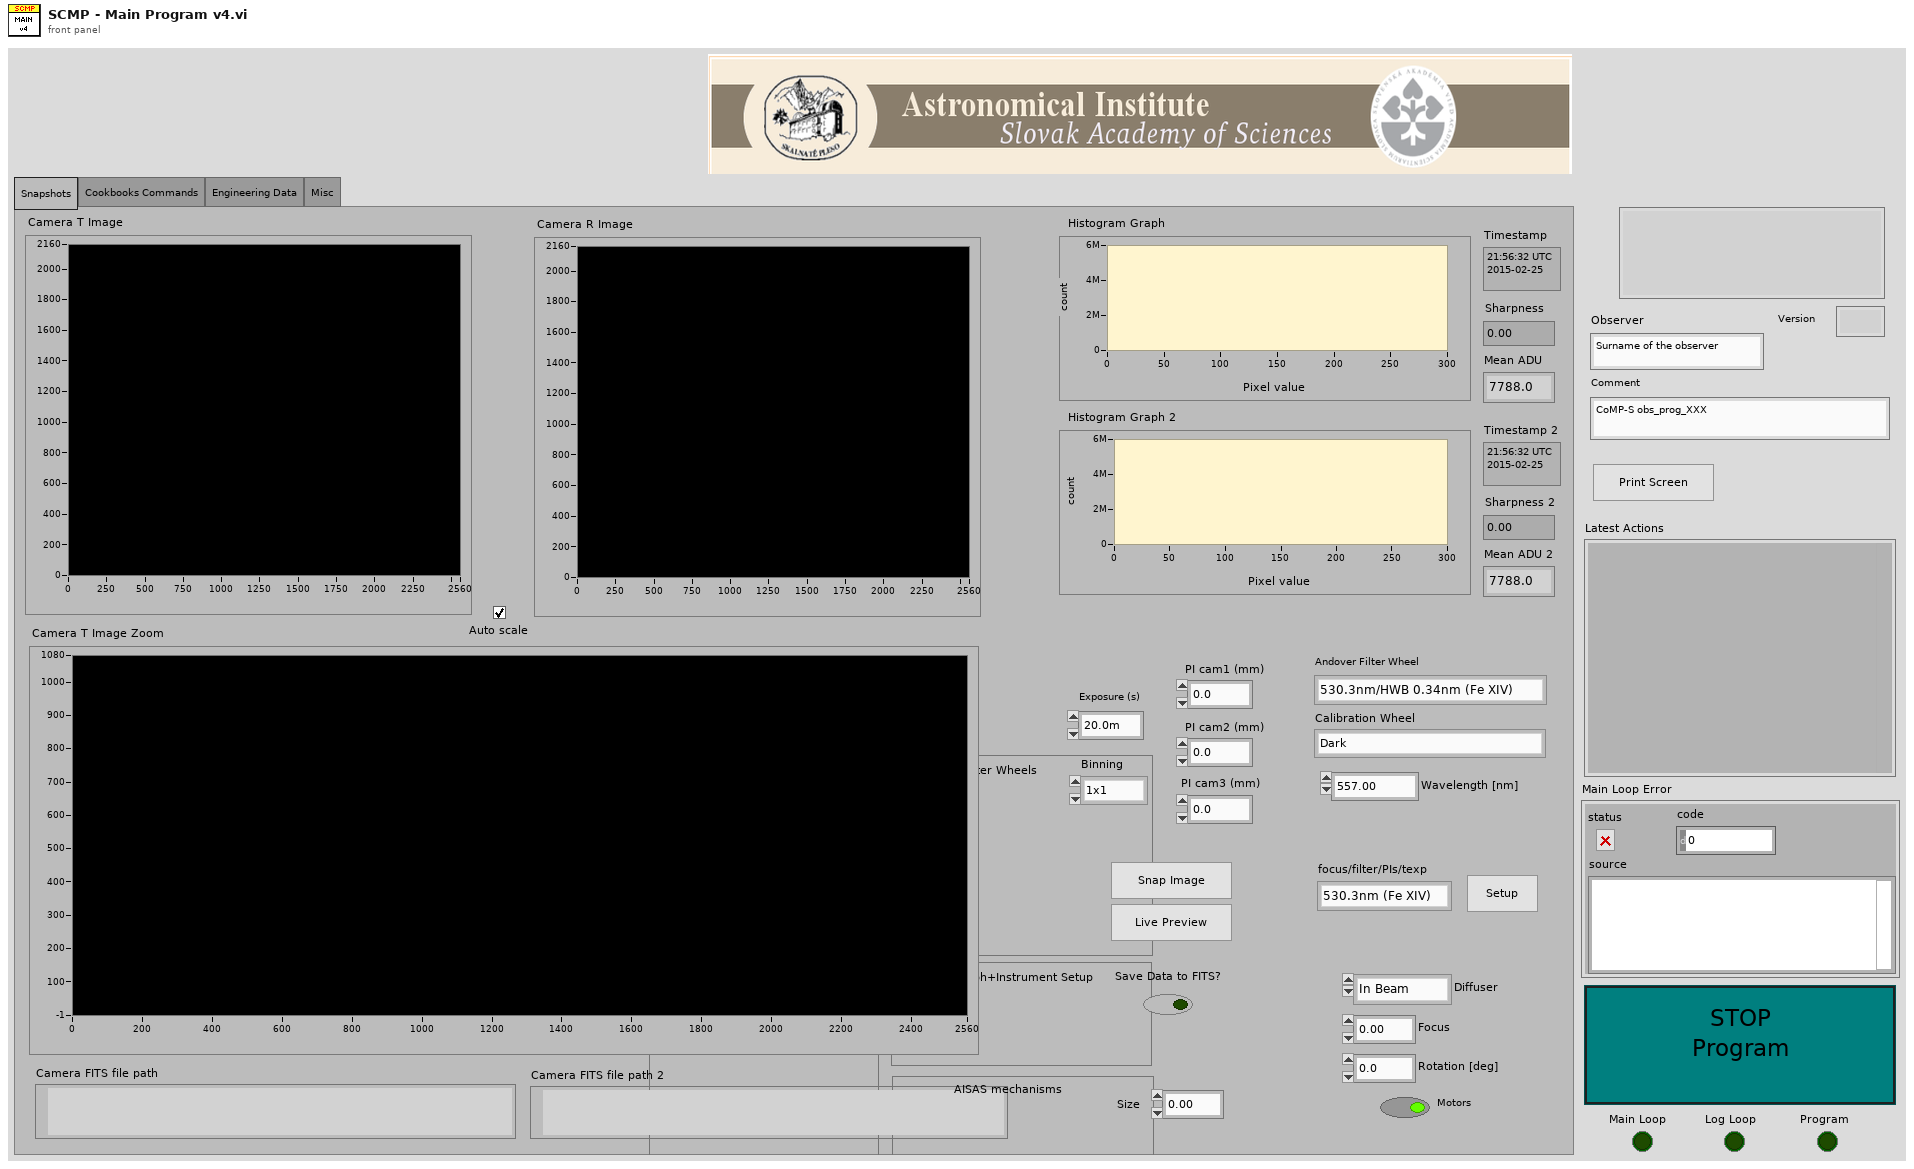
[diagram p1: front panel]
types:
  T1 = enum32{"Snapshots", "Cookbooks Commands", "Engineering Data", "Misc"}
  T2 = cluster{"X Values":dbl[], "Histogram: h(x)":i32[]}
  T3 = typedef "PI Control.ctl" = dbl
  T4 = typedef "SCD - Calibration Optics Filter Wheel.ctl" = enum16{"1 - Polarizer @0, I+Q", "2 - Polarizer @90, I-Q", "3 - Polarizer @45, I+U", "4 - Polarizer @135, I-U", "5 - Polarizer @0, Retarder @45, I+V", "6 - Polarizer @0, Retarder @135, I-V", "7 - Dark", "8 - Clear", "9 - N/A"}
  T5 = typedef "focus.ctl" = dbl
  T6 = typedef "Emission Line Filter Wheel.ctl" = enum16{"530.3nm/HWB 0.34nm (Fe XIV)", "587.6nm/HBW 0.44nm (He I D3)", "637.5nm/HBW 0.53nm (Fe X)", "656.3nm/HBW 0.57nm (H-Alpha)", "789.2nm/HBW 0.85nm (Fe XI)", "854.2nm/HBW 1.01nm (Ca I)", "1074.7nm/HBW 2.34nm (Fe XIII)", "1079.8nm/HBW 1.64nm (Fe XIII)", "1083.0nm/HBW 1.66nm (He I)"}
  T7 = typedef "Polarization Optics Filter Wheel.ctl" = enum16{"Dark", "Clear", "Exchange Lens", "Polarizer @0, I+Q", "Polarizer @90, I-Q", "Polarizer @45, I+U", "Polarizer @135, I-U", "Polarizer @0, Retarder @45, I+V", "Polarizer @0, Retarder @135, I-V"}
  T8 = typedef "beaning.ctl" = enum16{"1x1", "2x2", "3x3", "4x4", "8x8"}
  T9 = typedef "SCD - EDT - Emission Line Filter Wheel.ctl" = enum16{"1-557.6nm", "2-587.6nm", "3-589.6nm", "4-630.2nm", "5-656.4nm", "6-849.8nm", "7-854.2nm", "8-866.2nm", "9-1083.0nm"}
  T10 = typedef "Diffuser.ctl" = enum16{"Out of Beam", "In Beam"}
  T11 = typedef "Rotation.ctl" = dbl
  T12 = typedef "Cameras select.ctl" = enum16{"Andor", "GDR"}
  T13 = typedef "Cookbook.ctl" = cluster{"Data Type":T14, "Arg 1":sgl, "Arg 2":sgl, "Arg 3":path, "Comments":string}[]
  T14 = typedef "Cbk Data type.ctl" = enum32{"ACQUIRE DATA", "SET DIFFUSER", "CAL-FW", "WAVELENGTH-FW", "INSTR. ROTATION", "SET FOCUS", "DATATYPE", "SET EXPOSURE", "CBK COMMENTS", "MOVE-PI", "MOVE-PI2", "MOVE-PI3", "DWELL TIME", "BINNING"}
  T15 = typedef "SCD - FITS Cluster.ctl" = cluster{"Wavelength (nm)":dbl, "Exposure (s)":dbl, "Tuning Delay (ms)":dbl, "Beam Type (-1/1)":dbl, "Tuning Voltages":dbl[], "Observer":string, "Light Shapping Diffuser":T10, "Comment":string, "Data Type":T16, "Mod Cycles":u16, "SCD Calibration Optics":T4, "SCD Emission Line Filter":T9, "Cookbook":string, "COMP-S Calibration Wheel":T7, "COMP-S Andover Filter Wheel":T6, "FOV Rotation (deg)":dbl, "Objective Lens Position (mm)":T5, "Occulter size":dbl, "Time End":timestamp, "Acc Exposure (s)":dbl, "Time Stamp Array":timestamp[], "Camera Serial Number":string[], "Camera Temp":dbl[], "Camera PI (mm)":dbl[], "Time Start":timestamp, "Peripherals":T17, "FITS paths":path[], "Cameras":T12, "load preset cbk":bool, "periodic check count":i32, "COMP-S Calibration Wheel 2":T7, "Calib":enum16{"Dark", "Flat"}, "Abso Aperture":dbl, "Nominal Aperture":dbl, "Pointer IP":string}
  T16 = typedef "FITS Data type.ctl" = enum16{"LIVE", "DARK", "FLAT", "CALI", "OBSE", "ABSO", "AURE", "TARG", "OBJE", "HOLE", "OREX", "THRO", "CHIP"}
  T17 = typedef "peripherals.ctl" = cluster{"ILX controler":bool, "Zone temperatures":bool, "Andor":bool, "Andor 2":bool, "PI Stages":bool, "AISAS mechanisms":bool, "AISAS Mech.lvclass":refnum<class "AISAS Mech.lvclass">, "Zone temp ref":variant, "FWs":bool}
  T18 = typedef "Main Program States.ctl" = enum16{"Initialize", "Wait for Event", "Periodic Check", "Update UI", "Update Camera UI", "Load Cookbook", "Run Cookbook", "Snap Images", "Live Preview", "Set Filter Wheel", "Set Calibration Wheel", "AISAS Motors on/off", "AISAS Move", "Move AISAS Mechanisms", "Stop", "Change Camera Exposure", "Change Camera Stage Position", "Set Camera AOI", "Andor Adv Settings", "Update Image", "Run Dark", "Calib acq", "Process Calib"}
  T19 = enum8{"Enabled", "Disabled", "Disabled and Grayed Out"}
  T20 = typedef "pR Variable References.ctl" = cluster{"pLV":refnum<k21>, "COMPs":refnum<k21>, "Disable loopback":refnum<k21>}
  T21 = cluster{"Image Data Arr":u32[][][], "Dark":u32[][], "Flat":u32[][]}
  T22 = enum32{"Invalid", "Standard", "Closed", "Hidden", "Minimized", "Maximized"}
  T23 = typedef "motor.ctl" = enum32{"Rotation", "Diffuser ", "Focus"}
  T24 = enum16{"Emission Line Filters", "Calibration Polarizers"}
  T25 = typedef "imagedata.ctl" = cluster{"image type":i32, "image depth":i32, "image":u8[], "mask":u8[], "colors":u32[], "Rectangle":cluster{"left":i16, "top":i16, "right":i16, "bottom":i16}}
  T26 = typedef "DialogType.ctl" = u16
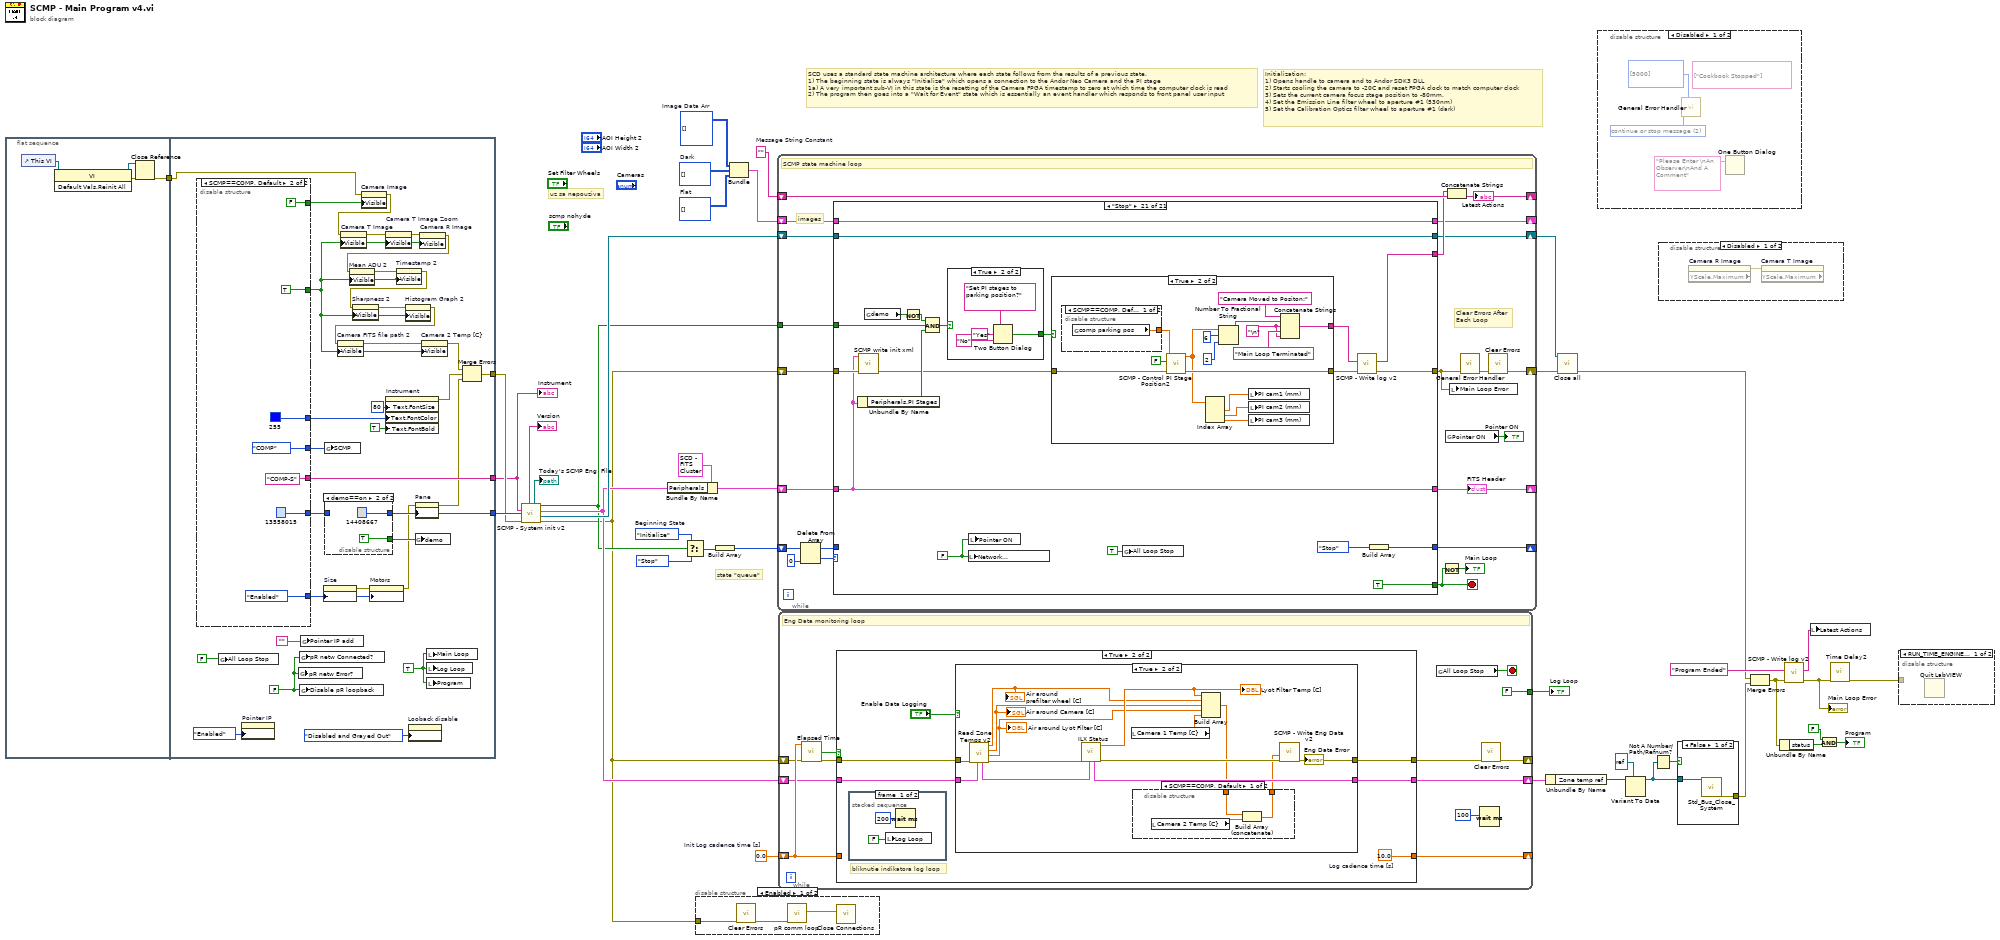
[diagram p0: block diagram]
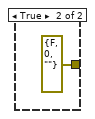
[diagram p5: hidden frame]
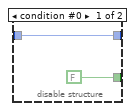
[diagram p6: hidden frame]
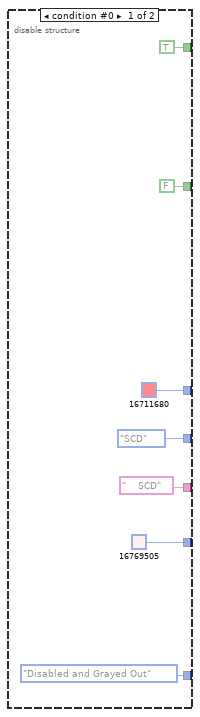
[diagram p7: hidden frame]
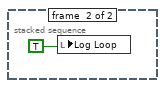
[diagram p10: hidden frame]
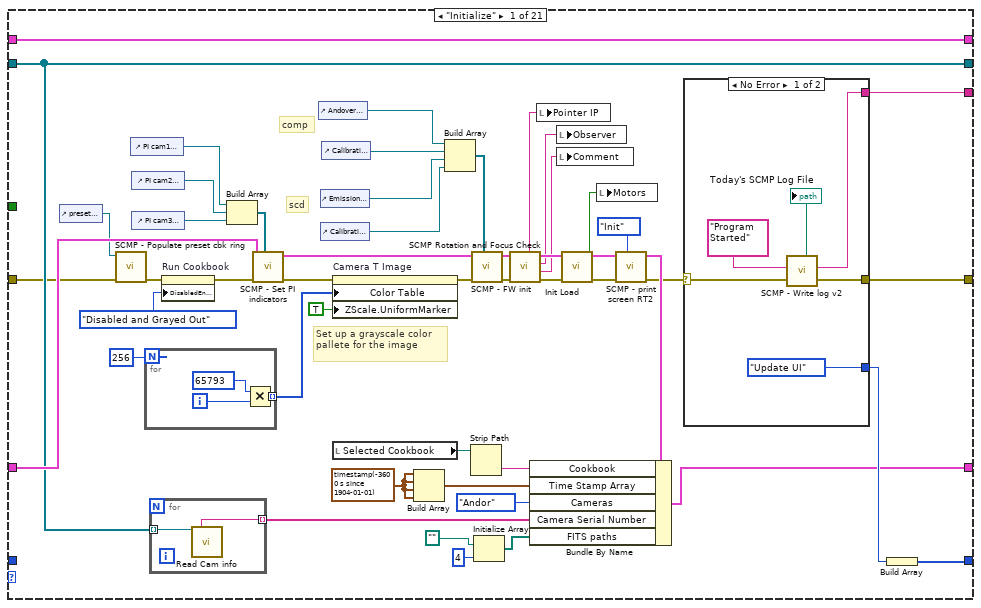
[diagram p13: hidden frame]
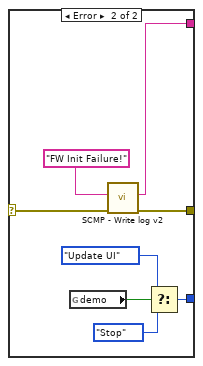
[diagram p14: hidden frame]
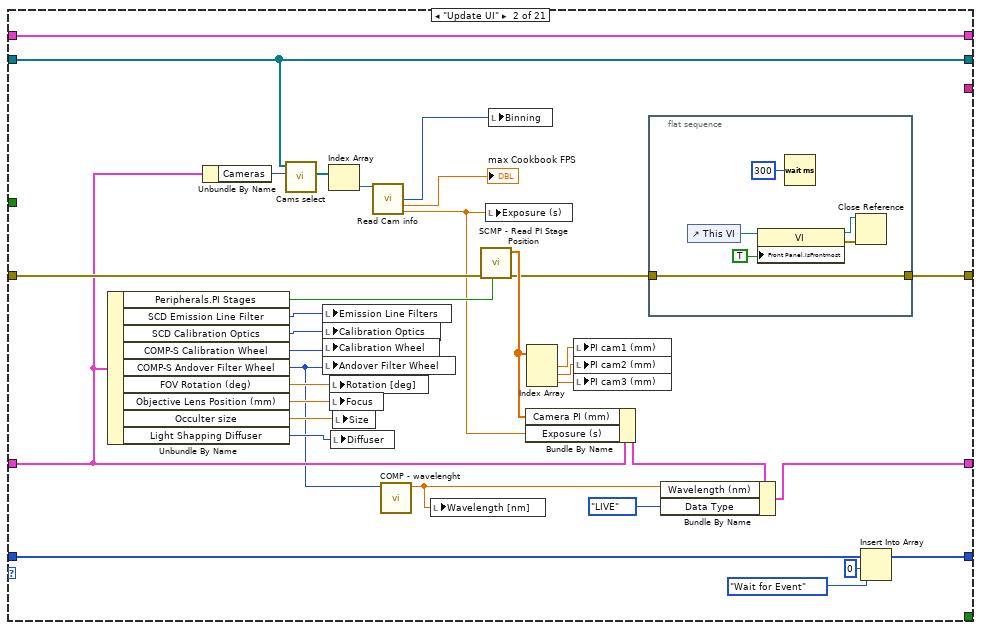
[diagram p15: hidden frame]
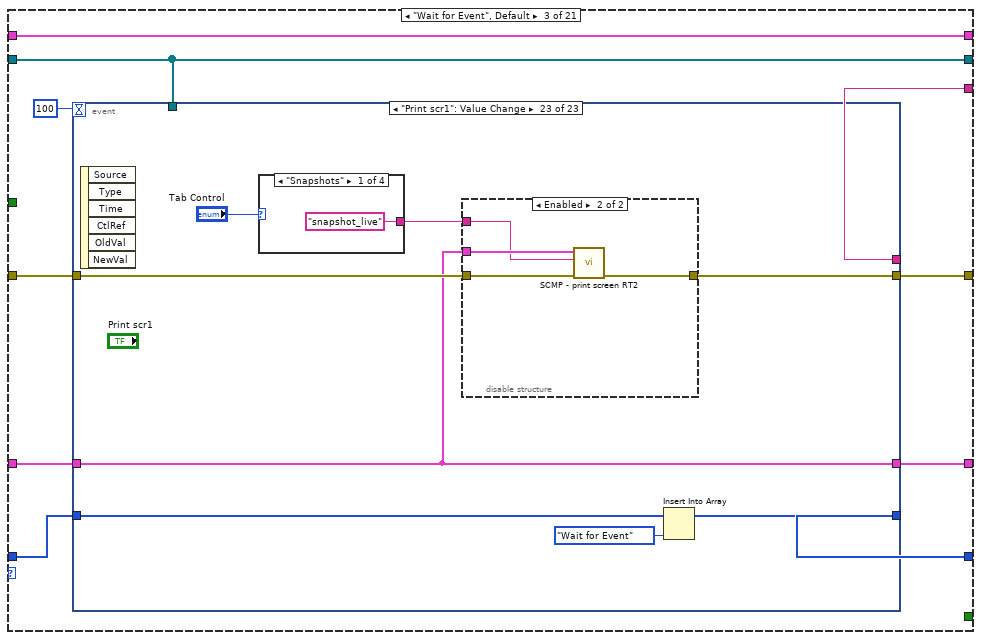
[diagram p16: hidden frame]
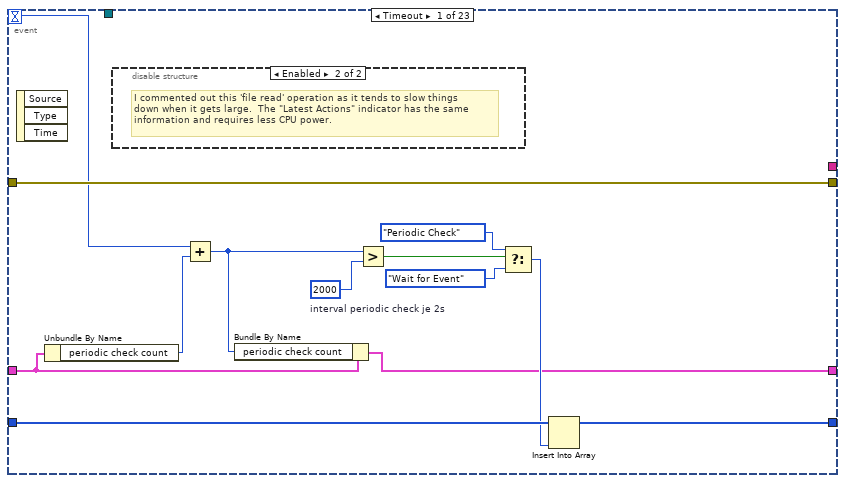
[diagram p17: hidden frame]
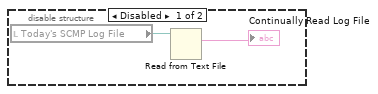
[diagram p18: hidden frame]
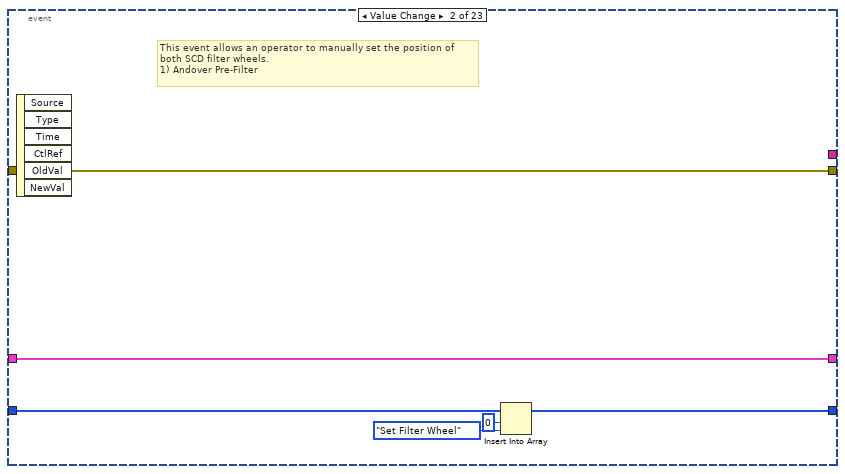
[diagram p19: hidden frame]
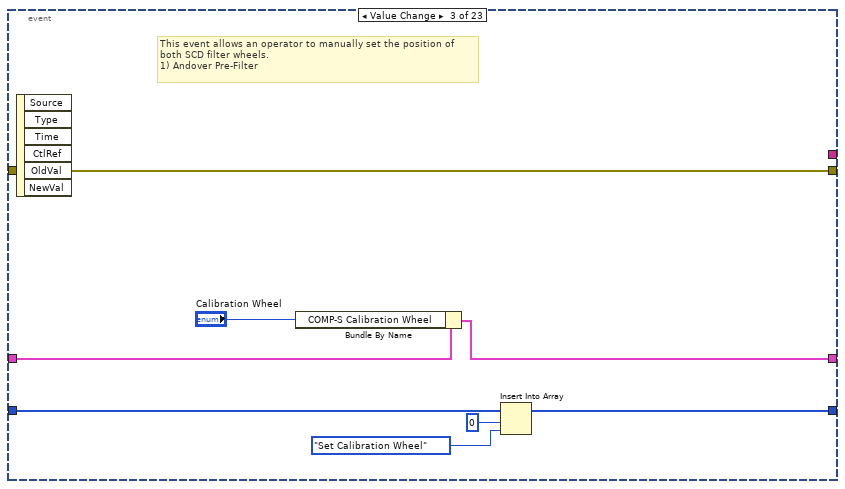
[diagram p20: hidden frame]
diagram:
  w8 = u32[][] []  # Flat
  w10 = u32[][] []  # Dark
  w11 = u32[][][] []  # Image Data Arr
  w24 = Main_Program_States."Initialize"  # Beginning State
  w38 = 0.0  # Init Log cadence time [s]
  w40 = ""  # Message String Constant
  # "state \"queue\""
  # "uz sa nepouziva"
  # "Initialization:\n1) Opens handle to camera and to Andor SDK3 DLL\n2) Starts cooling the camera to -20C and reset FPGA clock to match computer clock\n3) Sets the current camera focus stage position to -80mm.\n4) Set the Emission Line filter wheel to aperture #1 (530nm)\n5) Set the Calibration Optics filter wheel to aperture #1 (dark)"
  # "SCD uses a standard state machine architecture where each state follows from the results of a previous state.\n1) The beginning state is always \"Initialize\" which opens a connection to the Andor Neo Camera and the PI stage\n1a) A very important sub-VI in this state is the resetting of the Camera FPGA timestamp to zero at which time the computer clock is read\n2) The program then goes into a \"Wait for Event\" state which is essentially an event handler which responds to front panel user input"
  n1 = flat-sequence {
    tunnel: [w41] -> w12
    tunnel: [w68] -> w26
    tunnel: [w67] -> w20
    tunnel: [w54] -> w25
    tunnel: w12 -> [w50]
    frame #0 {
      n2 = control-ref of="This VI"() -> (w42:refnum<vi>)
      n3 = invoke class="VI" method="Default Vals.Reinit All"(reference=w42) -> (reference out=w44:refnum<vi>, error out=w43:errorcluster)  [unwired: 2 in, 1 out]
      n4 = Close Reference(reference=w44, error in (no error)=w43) -> (error out=w41:errorcluster)
    }
    frame #1 {
      w48 = FALSE ("All Loop Stop")
      w51 = TRUE ("Log Loop")
      n5 = disable-structure "Conditional Disable Structure" shown="SCMP==COMP, Default" {
        disable-tunnel: [TRUE ("Visible") FALSE ("Visible")] -> w72
        disable-tunnel: ["    SCD" ("String") "COMP-S" ("String")] -> w67
        disable-tunnel: [u32 16711680 u32 255] -> w75
        disable-tunnel: [u32 16769505 u32 13558015] -> w74
        disable-tunnel: [T19."Disabled and Grayed Out" ("Disabled") T19."Enabled" ("Disabled")] -> w70
        disable-tunnel: [FALSE ("Visible") TRUE ("Visible")] -> w69
        disable-tunnel: [enum16{"COMP", "SCD"}."SCD" ("SCMP") enum16{"COMP", "SCD"}."COMP" ("SCMP")] -> w71
        frame condition #0 {
        }
        frame condition #1 (active) {
        }
      }
      n6 = global write "Global - All Loop Stop.vi" "All Loop Stop"(FALSE ("All Loop Stop")) -> ()
      n7 = property on="Pointer IP" class="Str"("DisabledEnum"=T19."Enabled" ("Disabled")) -> ()  [unwired: 2 in, 2 out]
      n8 = global write "Global - pR netw comm.vi" "pR netw Error?"(w48) -> ()
      n9 = global write "Global - pR netw comm.vi" "pR netw Connected?"(w48) -> ()
      n10 = global write "Global - pR netw comm.vi" "Disable pR loopback"(w48) -> ()
      n11 = global write "Global - pR netw comm.vi" "Pointer IP add"("") -> ()
      n12 = property on="Size" class="DigNum (strict)"("DisabledEnum"=w70) -> (error out=w66:errorcluster)  [unwired: 2 in, 1 out]
      n13 = global write "Globals.vi" "SCMP"(w71) -> ()
      n14 = disable-structure shown="demo==on" {
        disable-tunnel: [w79 u32 14408667] -> w68
        disable-tunnel: w74 -> [w79 _]
        disable-tunnel: [FALSE ("demo") TRUE ("demo")] -> w73
        frame condition #0 {
        }
        frame condition #1 (active) {
        }
      }
      n15 = property on="Camera Image" class="IntGraph (strict)"(error in=w50, "Visible"=w72) -> (error out=w56:errorcluster)  [unwired: 1 in, 1 out]
      n16 = property on="Camera T Image" class="IntGraph (strict)"(error in=w56, "Visible"=w69) -> (error out=w62:errorcluster)  [unwired: 1 in, 1 out]
      n17 = property on="Motors" class="Bool (strict)"(error in=w66, "DisabledEnum"=w70) -> (error out=w65:errorcluster)  [unwired: 1 in, 1 out]
      n18 = property on="Camera T Image Zoom" class="IntGraph (strict)"(error in=w62, "Visible"=w69) -> (error out=w61:errorcluster)  [unwired: 1 in, 1 out]
      n19 = property on="Instrument" class="Str"("Text.FontSize"=u32 80 ("Text.Font:Color"), "Text.FontColor"=w75, "Text.FontBold"=TRUE ("Text.Font:Bold")) -> (error out=w53:errorcluster)  [unwired: 2 in, 1 out]
      n20 = property on="Looback disable" class="Bool (strict)"("DisabledEnum"=T19."Disabled and Grayed Out" ("Disabled")) -> ()  [unwired: 2 in, 2 out]
      n21 = property on="Pane" class="Pane"(error in=w65, "PaneColor"=w68) -> (error out=w52:errorcluster)  [unwired: 1 in, 1 out]
      n22 = global write "Global demo.vi" "demo"(w73) -> ()
      n23 = property on="Camera R Image" class="IntGraph (strict)"(error in=w61, "Visible"=w69) -> (error out=w60:errorcluster)  [unwired: 1 in, 1 out]
      n24 = property on="Mean ADU 2" class="DigNum (strict)"(error in=w60, "Visible"=w69) -> (error out=w59:errorcluster)  [unwired: 1 in, 1 out]
      n25 = property on="Timestamp 2" class="AbsTime (strict)"(error in=w59, "Visible"=w69) -> (error out=w58:errorcluster)  [unwired: 1 in, 1 out]
      n26 = property on="Sharpness 2" class="DigNum (strict)"(error in=w58, "Visible"=w69) -> (error out=w57:errorcluster)  [unwired: 1 in, 1 out]
      n27 = property on="Histogram Graph 2" class="XYGraph (strict)"(error in=w57, "Visible"=w69) -> (error out=w63:errorcluster)  [unwired: 1 in, 1 out]
      n28 = property on="Camera FITS file path 2" class="Path"(error in=w63, "Visible"=w69) -> (error out=w64:errorcluster)  [unwired: 1 in, 1 out]
      n29 = property on="Camera 2 Temp [C}" class="WFChart (strict)"(error in=w64, "Visible"=w69) -> (error out=w55:errorcluster)  [unwired: 1 in, 1 out]
      n30 = local write "Main Loop"(w51) -> ()
      n31 = local write "Log Loop"(w51) -> ()
      n32 = local write "Program"(w51) -> ()
      n33 = Merge Errors(w55, w53, w52) -> (w54:errorcluster)
    }
  }
  n34 = call "SCMP - System init v2.vi"("error in (no error)"=w25, "Pane Color"=w26, "instrument"=w20) -> ("error main"=w6:errorcluster, "Cameras"=w29:refnum<class "Camera.lvclass">[], "Peripherals"=w28:T17, "cont?"=w22:bool, "Today's SCMP Engineering File"=→"Today's SCMP Eng  File":path, "Version"=→"Version":string)  [unwired: 3 in]
  n35 = Bundle By Name(cluster=T15 {"Wavelength (nm)"=530.15, "Exposure (s)"=0.05, "Tuning Delay (ms)"=200.0, "Beam Type (-1/1)"=1.0, "Tuning Voltages"=[1.111, 2.222, 3.333, 4.444], "Observer"="observer", "Light Shapping Diffuser"=enum."In Beam", "Comment"="", "Data Type"=enum."LIVE", "Mod Cycles"=1, "SCD Calibration Optics"=enum."1 - Polarizer @0, I+Q", "SCD Emission Line Filter"=enum."1-557.6nm", "Cookbook"="", "COMP-S Calibration Wheel"=enum."Dark", "COMP-S Andover Filter Wheel"=enum."530.3nm/HWB 0.34nm (Fe XIV)", "FOV Rotation (deg)"=66.0, "Objective Lens Position (mm)"=0.0, "Occulter size"=0.0, "Time End"=timestamp(3382374145.421875 s since 1904-01-01), "Acc Exposure (s)"=0.0, "Time Stamp Array"=[], "Camera Serial Number"=[], "Camera Temp"=[], "Camera PI (mm)"=[0.0, 0.0, 0.0], "Time Start"=timestamp(3382374145.421875 s since 1904-01-01), "Peripherals"={"ILX controler"=FALSE, "Zone temperatures"=FALSE, "Andor"=FALSE, "Andor 2"=FALSE, "PI Stages"=FALSE, "AISAS mechanisms"=FALSE, "AISAS Mech.lvclass"=refnum, "Zone temp ref"=variant, "FWs"=FALSE}, "FITS paths"=[], "Cameras"=enum."Andor", "load preset cbk"=FALSE, "periodic check count"=0, "COMP-S Calibration Wheel 2"=enum."Dark", "Calib"=enum."Dark", "Abso Aperture"=66.0, "Nominal Aperture"=66.0, "Pointer IP"="127.0.0.1"} ("FITS"), "Peripherals"=w28) -> (w31:T15)
  n36 = Select(t=w24, s=w22, f=Main_Program_States."Stop" ("Beginning State")) -> (s? t:f=w14:T18)
  n37 = disable-structure shown="Enabled" {
    disable-tunnel: w6 -> [w98 _]
    frame Enabled {
      n38 = call <vilib>:"Clear Errors.vi"("error in (no error)"=w98) -> ("error out"=w97:errorcluster)  [unwired: 5 in, 1 out]
      n39 = call "pR comm loop.vi"("error in (no error)"=w97) -> ("netw Variable References"=w96:T20)  [unwired: 10 in]
      n40 = call "Close Connections.vi"("netw Variable References"=w96) -> ()  [unwired: 11 in]
    }
    frame Disabled {
    }
  }
  n41 = Build Array(w14) -> (w13:T18[])
  n42 = Bundle("Image Data Arr"=w11, "Dark"=w10, "Flat"=w8) -> (w9:T21)  [unwired: 1 in]
  n43 = while {
    shift-right: [w114] -> w5
    shift-left: w6 -> [w120]
    shift-right: [w115] -> _
    shift-left: w40 -> [w117]
    shift-right: [w109] -> _
    shift-left: w31 -> [w119]
    shift-right: [w110] -> w15
    shift-left: w29 -> [w118]
    shift-right: [w102] -> _
    shift-left: w13 -> [w105]
    tunnel: w22 -> [w108]
    shift-right: [w107] -> _
    shift-left: w9 -> [w106]
    stop <- w100 stop-if-true
    # "images"
    # "Clear Errors After\nEach Loop"
    # "SCMP state machine loop"
    n44 = Delete From Array(array=w105, index=0) -> (deleted portion=w104:T18, array with subset deleted=w103:T18[])  [unwired: 1 in]
    n45 = case shown="\"Stop\"" w104 {
      tunnel: w120 -> [w135 w217 w237 w486 w517 w575 w585 w640 w679 w737 w766 w797 w826 w858 w894 w912 w946 w959 w973 w1000 w1025]
      tunnel: [w170 w205 w236 w464 w519 w569 w580 w638 w681 w735 w765 w796 w812 w855 w893 w918 w939 w958 w969 w999 w1038] -> w111
      tunnel: [w165 _ w232 w467 _ w568 _ w648 w697 w739 w768 w795 w828 w859 w895 w919 _ _ _ _ w1040] -> w116
      tunnel: w119 -> [w152 w210 w235 w487 w522 w573 w583 w617 w714 w731 w761 w792 w827 w849 w889 w906 w945 w965 w981 w1002 w1023]
      tunnel: [w129 w191 w234 w473 w522 w567 w581 w647 w703 w730 w760 w791 w811 w856 w889 w906 w945 w963 w976 w1006 w1023] -> w109
      tunnel: w118 -> [w142 w209 w229 w478 w524 w574 w584 w620 w693 w738 w767 w805 w831 w857 w885 w913 w935 w966 w993 w1007 w1039]
      tunnel: [w142 w209 w229 w478 w524 w572 w582 w620 w692 w738 w767 w805 w831 w857 w884 w910 w934 w966 w992 w1007 w1039] -> w110
      tunnel: [_ _ _ _ _ _ _ _ _ _ _ _ _ _ _ _ _ _ _ _ TRUE ("x = y?")] -> w100
      tunnel: w108 -> [_ _ _ _ _ _ _ _ _ _ _ _ _ _ _ _ _ _ _ _ w1029]
      tunnel: [w143 w214 w233 w479 w518 w558 w577 w634 w694 w728 w759 w789 w810 w845 w892 w916 w944 w967 w990 w1003 w1028] -> w107
      tunnel: w106 -> [w143 w214 w233 w479 w518 w560 w578 w634 w694 w728 w759 w789 w810 w845 w892 w916 w944 w967 w991 w1004 w1028]
      tunnel: w103 -> [_ w202 w231 _ w520 w565 _ w633 w691 w727 w758 w788 w809 w844 w878 w905 w932 _ w982 w998 _]
      tunnel: [w137 w203 w230 w471 w520 w564 w576 w632 w690 w726 w757 w787 w808 w843 w877 w904 w931 w960 w982 w1005 w1026] -> w102
      frame "Initialize" {
        w166 = timestamp(-3600 s since 1904-01-01) ("element")
        # "Set up a grayscale color pallete for the image"
        # "scd"
        # "comp"
        n46 = control-ref of="preset cbk"() -> (w134:refnum<vi>)
        n47 = call "SCMP - Populate preset cbk ring.vi"("error in (no error)"=w135, "preset cbk ring ref"=w134) -> ("error out"=w133:errorcluster)  [unwired: 9 in]
        n48 = control-ref of="PI cam1 (mm)"() -> (w154:refnum<vi>)
        n49 = control-ref of="PI cam2 (mm)"() -> (w155:refnum<vi>)
        n50 = control-ref of="PI cam3 (mm)"() -> (w156:refnum<vi>)
        n51 = for {
          N: 256 -> [_]
          tunnel: [w174] -> w149 mode=indexing
          i -> [w175]
          n52 = Multiply(x=65793, y=w175) -> (x*y=w174:i32)
        }
        n53 = for {
          tunnel: w142 -> [w172] mode=indexing
          tunnel: [w171] -> w141 mode=indexing
          n54 = call-dynamic "Read Cam info.vi"("Camera in"=w172) -> ("SerialNumber"=w171:string)  [unwired: 5 in, 9 out]
        }
        n55 = property on="Run Cookbook" class="Bool"(error in=w133, "DisabledEnum"=T19."Disabled and Grayed Out" ("Disabled")) -> (error out=w132:errorcluster)  [unwired: 1 in, 1 out]
        n56 = Build Array(w154, w155, w156) -> (w153:refnum<vi>[])
        n57 = call "SCMP - Set PI indicators.vi"("PI refs"=w153, "error in (no error)"=w132, "FITS Header in"=w152) -> ("error out"=w148:errorcluster, "FITS Header out"=w151:T15)  [unwired: 7 in]
        n58 = control-ref of="Andover Filter Wheel"() -> (w130:refnum<vi>)
        n59 = control-ref of="Emission Line Filters"() -> (w159:refnum<vi>)
        n60 = control-ref of="Calibration Optics"() -> (w158:refnum<vi>)
        n61 = control-ref of="Calibration Wheel"() -> (w160:refnum<vi>)
        n62 = property on="Camera T Image" class="IntGraph (strict)"(error in=w148, "Color Table"=w149, "ZScale.UniformMarker"=TRUE ("Z Scale.Uniform Marker Spacing?")) -> (error out=w147:errorcluster)  [unwired: 1 in, 1 out]
        n63 = local read "Selected Cookbook"() -> (w169:path)
        n64 = Build Array(w166, w166, w166, w166) -> (w145:timestamp[])
        n65 = Build Array(w130, w160, w159, w158) -> (w157:refnum<vi>[])
        n66 = Strip Path(path=w169) -> (name=w168:string)  [unwired: 1 out]
        n67 = call "SCMP - FW init.vi"("FW refs"=w157, "error in (no error)"=w147, "FITS Header in"=w151) -> ("error out"=w167:errorcluster, "FITS Header out"=w163:T15)  [unwired: 7 in]
        n68 = Initialize Array(path "", 4 ("dimension size")) -> (w138:path[])
        n69 = call "SCMP Rotation and Focus Check.vi"("error in"=w167, "FITS Header In"=w163) -> ("error out"=w164:errorcluster, "Comment out"=w127:string, "Observer out"=w128:string, "FITS Header Out"=w162:T15, "Pointer IP"=w121:string)  [unwired: 5 in]
        n70 = local write "Pointer IP"(w121) -> ()
        n71 = local write "Observer"(w128) -> ()
        n72 = local write "Comment"(w127) -> ()
        n73 = call "Init Load.vi"("error in (no error)"=w164, "FITS Header in"=w162) -> ("error out"=w126:errorcluster, "Motors (off/on)"=w161:bool, "FITS Header out"=w125:T15)  [unwired: 7 in]
        n74 = local write "Motors"(w161) -> ()
        n75 = call "SCMP - print screen RT2.vi"("mode (save)"=enum16{"Init", "Save"}."Init", "error in (no error)"=w126, "FITS Header in"=w125) -> ("error out"=w123:errorcluster, "FITS Header out"=w124:T15)  [unwired: 7 in]
        n76 = Bundle By Name(cluster=w124, "Cookbook"=w168, "Time Stamp Array"=w145, "Cameras"=Cameras_select."Andor", "Camera Serial Number"=w141, "FITS paths"=w138) -> (w129:T15)
        n77 = case shown="No Error" w123 {
          selector: w123 -> [w179 w189]
          tunnel: [w177 w186] -> w165
          tunnel: [w178 w188] -> w170
          tunnel: [Main_Program_States."Update UI" ("Beginning State") w182] -> w136
          frame No Error {
            n78 = call "SCMP - Write log v2.vi"("Error to log"=w179, "data"="Program Started") -> ("error out"=w178:errorcluster, "Last Log Entry"=w177:string, "Today's SCMP Log File"=→"Today's SCMP Log File":path)  [unwired: 7 in]
          }
          frame Error {
            n79 = global read "Global demo.vi" "demo"() -> (w183:bool)
            n80 = call "SCMP - Write log v2.vi"("Error to log"=w189, "data"="FW Init Failure!") -> ("error out"=w188:errorcluster, "Last Log Entry"=w186:string)  [unwired: 7 in, 1 out]
            n81 = Select(t=Main_Program_States."Update UI" ("Beginning State"), s=w183, f=Main_Program_States."Stop" ("Beginning State")) -> (s? t:f=w182:T18)
          }
        }
        n82 = Build Array(w136) -> (w137:T18[])
      }
      frame "Update UI" {
        n83 = Unbundle By Name(w210) -> ("Peripherals.PI Stages"=w216:bool, "SCD Emission Line Filter"=w218:T9, "SCD Calibration Optics"=w219:T4, "COMP-S Calibration Wheel"=w193:T7, "COMP-S Andover Filter Wheel"=w192:T6, "FOV Rotation (deg)"=w201:dbl, "Objective Lens Position (mm)"=w200:T5, "Occulter size"=w199:dbl, "Light Shapping Diffuser"=w194:T10)
        n84 = Unbundle By Name(w210) -> ("Cameras"=w213:T12)
        n85 = call "Cams select.vi"("Cameras"=w213, "Cameras in"=w209) -> ("Cams selection"=w212:refnum<class "Camera.lvclass">[])  [unwired: 8 in, 1 out]
        n86 = local write "Emission Line Filters"(w218) -> ()
        n87 = local write "Calibration Optics"(w219) -> ()
        n88 = local write "Calibration Wheel"(w193) -> ()
        n89 = local write "Andover Filter Wheel"(w192) -> ()
        n90 = Index Array(array=w212) -> (element=w211:refnum<class "Camera.lvclass">)  [unwired: 1 in]
        n91 = local write "Rotation [deg]"(w201) -> ()
        n92 = local write "Focus"(w200) -> ()
        n93 = local write "Diffuser"(w194) -> ()
        n94 = local write "Size"(w199) -> ()
        n95 = call-dynamic "Read Cam info.vi"("Camera in"=w211) -> ("Binning"=w207:T8, "FPS"=→"max Cookbook FPS":dbl, "Exposure [s]"=w208:dbl)  [unwired: 5 in, 7 out]
        n96 = call "COMP - wavelenght.vi"("COMP-S Andover Filter Wheel"=w192) -> ("Wavelength (nm)"=w195:dbl)  [unwired: 10 in]
        n97 = local write "Wavelength [nm]"(w195) -> ()
        n98 = call "SCMP - Read PI Stage Position.vi"("Enable"=w216, "error in (no error)"=w217) -> ("error out"=w206:errorcluster, "Output Array"=w215:dbl[])  [unwired: 8 in]
        n99 = local write "Exposure (s)"(w208) -> ()
        n100 = local write "Binning"(w207) -> ()
        n101 = Bundle By Name(cluster=w210, "Camera PI (mm)"=w215, "Exposure (s)"=w208) -> (w196:T15)
        n102 = Index Array(array=w215) -> (element #1=w220:dbl, element #2=w221:dbl, element #3=w222:dbl)  [unwired: 3 in]
        n103 = local write "PI cam1 (mm)"(w220) -> ()
        n104 = local write "PI cam2 (mm)"(w221) -> ()
        n105 = local write "PI cam3 (mm)"(w222) -> ()
        n106 = flat-sequence {
          tunnel: w206 -> [w224]
          tunnel: [w224] -> w205
          frame #0 {
            n107 = control-ref of="This VI"() -> (w225:refnum<vi>)
            n108 = property class="VI"(reference=w225, "Front Panel.IsFrontmost"=TRUE ("Front Panel Window:Is Frontmost")) -> (reference out=w228:refnum<vi>, error out=w227:errorcluster)  [unwired: 1 in]
            n109 = Wait (ms)(milliseconds to wait=u32 300) -> ()  [unwired: 1 out]
            n110 = Close Reference(reference=w228, error in (no error)=w227) -> ()  [unwired: 1 out]
          }
        }
        n111 = Bundle By Name(cluster=w196, "Wavelength (nm)"=w195, "Data Type"=FITS_Data_type."LIVE") -> (w191:T15)
        n112 = Insert Into Array(array=w202, index=0, new element=Main_Program_States."Wait for Event" ("Next State")) -> (w203:T18[])
      }
      frame "Wait for Event", Default {
        n113 = event shown="[22] \"Print scr1\": Value Change" {
          selector: _ -> [_ _ _ _ _ _ _ _ _ _ _ _ _ _ _ _ _ _ _ _ _ _ _]
          dyn-events: _ -> [_ _ _ _ _ _ _ _ _ _ _ _ _ _ _ _ _ _ _ _ _ _ _]
          timeout: 100 -> [w247 _ _ _ _ _ _ _ _ _ _ _ _ _ _ _ _ _ _ _ _ _ _]
          tunnel: w237 -> [w251 w259 w267 w273 w278 w282 w313 w320 w325 w331 w337 w350 w363 w376 w382 w388 w394 w400 w406 w421 w432 w438 w443]
          tunnel: [w251 w259 w267 w273 w278 w288 w313 w320 w325 w331 w337 w348 w361 w374 w382 w388 w394 w400 w406 w420 w431 w438 w441] -> w236
          tunnel: w235 -> [w241 w258 w262 w272 w277 w289 w312 w319 w324 w330 w336 w347 w360 w373 w381 w387 w393 w399 w405 w408 w428 w437 w442]
          tunnel: [w239 w258 w261 w272 w277 w289 w312 w317 w324 w330 w336 w345 w358 w371 w381 w387 w393 w399 w405 w408 w427 w437 w442] -> w234
          tunnel: [_ _ _ _ _ w287 _ _ _ _ _ _ _ _ _ _ _ _ _ _ _ _ _] -> w232
          tunnel: w231 -> [w250 w257 w266 w271 _ w286 _ _ _ w329 w335 w341 w354 w367 w380 w386 w392 w398 w404 w422 w425 w435 w445]
          tunnel: [w249 w256 w265 w270 w274 w285 w309 w316 w321 w328 w334 w340 w353 w366 w379 w385 w391 w397 w403 w422 w424 w434 w444] -> w230
          tunnel: w229 -> [_ _ _ _ _ _ _ _ _ _ _ _ _ _ _ _ _ _ _ w409 _ _ _]
          event Timeout {
            w246 = 2000  # interval periodic check je 2s
            n114 = event-data() -> ()  [unwired: 1 in, 3 out]
            n115 = Unbundle By Name(w241) -> ("periodic check count"=w248:i32)
            n116 = disable-structure shown="Enabled" {
              frame Disabled {
                n117 = local read "Today's SCMP Log File"() -> (w253:path)
                n118 = Read from Text File(file (use dialog)=w253) -> (text=→"Continually Read Log File":string)  [unwired: 3 in, 3 out]
              }
              frame Enabled {
                # "I commented out this 'file read' operation as it tends to slow things\ndown when it gets large.  The \"Latest Actions\" indicator has the same\ninformation and requires less CPU power."
              }
            }
            n119 = Add(x=w247, y=w248) -> (x+y=w240:i32)
            n120 = Bundle By Name(cluster=w241, "periodic check count"=w240) -> (w239:T15)
            n121 = Greater?(x=w240, y=w246) -> (0:w244:bool)
            n122 = Select(t=Main_Program_States."Periodic Check" ("Next State"), s=w244, f=Main_Program_States."Wait for Event") -> (s? t:f=w242:T18)
            n123 = Insert Into Array(array=w250, new element=w242) -> (w249:T18[])  [unwired: 1 in]
          }
          event Value Change {
            # "This event allows an operator to manually set the position of\nboth SCD filter wheels.  \n1) Andover Pre-Filter"
            n124 = event-data() -> ()  [unwired: 1 in, 6 out]
            n125 = Insert Into Array(array=w257, index=0, new element=Main_Program_States."Set Filter Wheel" ("Next State")) -> (w256:T18[])
          }
          event Value Change {
            # "This event allows an operator to manually set the position of\nboth SCD filter wheels.  \n1) Andover Pre-Filter"
            n126 = event-data() -> ()  [unwired: 1 in, 6 out]
            n127 = Bundle By Name(cluster=w262, "COMP-S Calibration Wheel"="Calibration Wheel") -> (w261:T15)
            n128 = Insert Into Array(array=w266, index=0, new element=Main_Program_States."Set Calibration Wheel" ("Next State")) -> (w265:T18[])
          }
          event Value Change {
            n129 = event-data() -> ()  [unwired: 1 in, 2 out]
            n130 = Insert Into Array(array=w271, index=0, new element=Main_Program_States."Change Camera Stage Position" ("Next State")) -> (w270:T18[])
          }
          event "Snap Images": Value Change {
            # "zrusi sa pripadny live preview mod"
            # "This event snaps a single Andor Neo image (untriggered)"
            n131 = event-data() -> ()  [unwired: 1 in, 6 out]
            n132 = local write "Live Preview"(FALSE ("Live Preview")) -> ()
            n133 = Build Array(Main_Program_States."Snap Images" ("Next State")) -> (w274:T18[])
          }
          event "Live Preview": Value Change {
            n134 = event-data() -> ("NewVal"=w280:bool)  [unwired: 1 in, 5 out]
            n135 = case shown="True" w280 {
              tunnel: w282 -> [w291 w297]
              tunnel: [w291 w300] -> w281
              tunnel: ["Live Preview off" ("Last Log Entry") "Live Preview on" ("Last Log Entry")] -> w279
              frame False {
              }
              frame True {
                # "live je o chlp rychlejsie ak sa zatvori front panel"
                n136 = vi-ref "Camera.lvclass:Data Acquisition - v8.vi"() -> (w298:refnum<vi>)
                n137 = property class="VI"(reference=w298, error in=w297) -> (reference out=w292:refnum<vi>, error out=w293:errorcluster, "FP.State"=w296:T22)
                n138 = Equal?(x=w296, y=T22."Closed") -> (x = y?=w294:bool)
                n139 = case shown="False" w294 {
                  tunnel: [w303 w308] -> w300
                  tunnel: w293 -> [w302 w307]
                  tunnel: w292 -> [w301 w306]
                  frame False {
                    n140 = invoke class="VI" method="FP.Close"(reference=w301, error in=w302) -> (reference out=w304:refnum<vi>, error out=w305:errorcluster)  [unwired: 1 in, 1 out]
                    n141 = Close Reference(reference=w304, error in (no error)=w305) -> (error out=w303:errorcluster)
                  }
                  frame True {
                    n142 = Close Reference(reference=w306, error in (no error)=w307) -> (error out=w308:errorcluster)
                  }
                }
              }
            }
            n143 = Insert Into Array(array=w286, index=0, new element=Main_Program_States."Live Preview" ("Next State")) -> (w285:T18[])
            n144 = call "SCMP - Write log v2.vi"("Error to log"=w281, "data"=w279) -> ("error out"=w288:errorcluster, "Last Log Entry"=w287:string)  [unwired: 7 in, 1 out]
          }
          event "Load Cookbook": Value Change {
            # "zrusi sa pripadny live preview mod"
            # "This event lets an observer select a cookbook to 'run'"
            n145 = event-data() -> ()  [unwired: 1 in, 6 out]
            n146 = local write "Live Preview"(FALSE ("Live Preview")) -> ()
            n147 = Build Array(Main_Program_States."Load Cookbook" ("Next State")) -> (w309:T18[])
          }
          event "Setup Cor": Value Change {
            # "zrusi sa pripadny live preview mod"
            # "This event load preset cookbook"
            n148 = event-data() -> ()  [unwired: 1 in, 6 out]
            n149 = Bundle By Name(cluster=w319, "load preset cbk"=TRUE) -> (w317:T15)
            n150 = local write "Live Preview"(FALSE ("Live Preview")) -> ()
            n151 = Build Array(Main_Program_States."Load Cookbook" ("Next State")) -> (w316:T18[])
          }
          event "Run Cookbook": Value Change {
            # "zrusi sa pripadny live preview mod"
            # "This event runs a previously loaded cookbook sequence\nCookbooks can take many minutes to run..."
            n152 = event-data() -> ()  [unwired: 1 in, 6 out]
            n153 = local write "Live Preview"(FALSE ("Live Preview")) -> ()
            n154 = Build Array(Main_Program_States."Run Cookbook" ("Next State")) -> (w321:T18[])
          }
          event "Move AISAS Mechanisms": Value Change {
            n155 = event-data() -> ()  [unwired: 1 in, 2 out]
            n156 = Insert Into Array(array=w329, index=0, new element=Main_Program_States."Move AISAS Mechanisms" ("Next State")) -> (w328:T18[])
          }
          event "Motors": Value Change {
            n157 = event-data() -> ()  [unwired: 1 in, 2 out]
            n158 = Insert Into Array(array=w335, index=0, new element=Main_Program_States."AISAS Motors on/off" ("Next State")) -> (w334:T18[])
          }
          event Value Change {
            n159 = event-data() -> ()  [unwired: 1 in, 6 out]
            n160 = Unbundle By Name(w347) -> ("Peripherals.AISAS Mech.lvclass"=w349:refnum<class "AISAS Mech.lvclass">)
            n161 = To Variant(anything="Diffuser") -> (Variant=w344:variant)
            n162 = call "Write Move Motor.vi"("error in (no error)"=w350, "Desired Value"=w344, "Motor"=motor."Diffuser ", "AISAS Mech in"=w349) -> ("error out"=w348:errorcluster, "AISAS Mech out"=w346:refnum<class "AISAS Mech.lvclass">)  [unwired: 6 in]
            n163 = Bundle By Name(cluster=w347, "Peripherals.AISAS Mech.lvclass"=w346) -> (w345:T15)
            n164 = Insert Into Array(array=w341, index=0, new element=Main_Program_States."AISAS Move" ("Next State")) -> (w340:T18[])
          }
          event Value Change {
            n165 = event-data() -> ()  [unwired: 1 in, 6 out]
            n166 = Unbundle By Name(w360) -> ("Peripherals.AISAS Mech.lvclass"=w362:refnum<class "AISAS Mech.lvclass">)
            n167 = To Variant(anything="Rotation [deg]") -> (Variant=w357:variant)
            n168 = call "Write Move Motor.vi"("error in (no error)"=w363, "Desired Value"=w357, "Motor"=motor."Rotation", "AISAS Mech in"=w362) -> ("error out"=w361:errorcluster, "AISAS Mech out"=w359:refnum<class "AISAS Mech.lvclass">)  [unwired: 6 in]
            n169 = Bundle By Name(cluster=w360, "Peripherals.AISAS Mech.lvclass"=w359) -> (w358:T15)
            n170 = Insert Into Array(array=w354, index=0, new element=Main_Program_States."AISAS Move" ("Next State")) -> (w353:T18[])
          }
          event Value Change {
            n171 = event-data() -> ()  [unwired: 1 in, 6 out]
            n172 = Unbundle By Name(w373) -> ("Peripherals.AISAS Mech.lvclass"=w375:refnum<class "AISAS Mech.lvclass">)
            n173 = To Variant(anything="Focus") -> (Variant=w370:variant)
            n174 = call "Write Move Motor.vi"("error in (no error)"=w376, "Desired Value"=w370, "Motor"=motor."Focus", "AISAS Mech in"=w375) -> ("error out"=w374:errorcluster, "AISAS Mech out"=w372:refnum<class "AISAS Mech.lvclass">)  [unwired: 6 in]
            n175 = Bundle By Name(cluster=w373, "Peripherals.AISAS Mech.lvclass"=w372) -> (w371:T15)
            n176 = Insert Into Array(array=w367, index=0, new element=Main_Program_States."AISAS Move" ("Next State")) -> (w366:T18[])
          }
          event "Exposure (s)": Value Change {
            n177 = event-data() -> ()  [unwired: 1 in, 2 out]
            n178 = Insert Into Array(array=w380, index=0, new element=Main_Program_States."Change Camera Exposure" ("Next State")) -> (w379:T18[])
          }
          event Value Change {
            n179 = event-data() -> ()  [unwired: 1 in, 3 out]
            n180 = Insert Into Array(array=w386, index=0, new element=Main_Program_States."Set Camera AOI" ("Next State")) -> (w385:T18[])
          }
          event "Andor Adv Settings": Value Change {
            n181 = event-data() -> ()  [unwired: 1 in, 2 out]
            n182 = Insert Into Array(array=w392, index=0, new element=Main_Program_States."Andor Adv Settings" ("Next State")) -> (w391:T18[])
          }
          event "Run Dark": Value Change {
            n183 = event-data() -> ()  [unwired: 1 in, 2 out]
            n184 = Insert Into Array(array=w398, index=0, new element=Main_Program_States."Run Dark" ("Next State")) -> (w397:T18[])
          }
          event "Stop": Value Change {
            # "This event causes the SCD program to terminate"
            n185 = event-data() -> ()  [unwired: 1 in, 1 out]
            n186 = Insert Into Array(array=w404, index=0, new element=Main_Program_States."Stop" ("Next State")) -> (w403:T18[])
          }
          event "Auto scale": Value Change {
            n187 = event-data() -> ("NewVal"=w407:bool)  [unwired: 1 in, 5 out]
            n188 = Unbundle By Name(w408) -> ("Cameras"=w411:T12)
            n189 = call "Cams select.vi"("Cameras"=w411, "Cameras in"=w409) -> ("Cams selection"=w410:refnum<class "Camera.lvclass">[])  [unwired: 8 in, 1 out]
            n190 = control-ref of="Camera T Image"() -> (w416:refnum<vi>)
            n191 = control-ref of="Camera R Image"() -> (w413:refnum<vi>)
            n192 = control-ref of="Camera T Image Zoom"() -> (w412:refnum<vi>)
            n193 = Index Array(array=w410) -> (element #1=w419:refnum<class "Camera.lvclass">)  [unwired: 2 in, 1 out]
            n194 = Build Array(w416, w413, w412) -> (w415:refnum<vi>[])
            n195 = Type Cast(type=refnum<vi>[] [] ("Ref Array"), x=w415) -> (*(type *) &x=w414:refnum<vi>[])
            n196 = call-dynamic "Read Cam info.vi"("Camera in"=w419) -> ("AOI Height"=w418:i32)  [unwired: 5 in, 9 out]
            n197 = call "Scale ui image graphs.vi"("AOI Height"=w418, "error in (no error)"=w421, "Auto scale"=w407, "Ref Array"=w414) -> ("error out"=w420:errorcluster)  [unwired: 7 in]
          }
          event "AISAS verification": Value Change {
            n198 = event-data() -> ("NewVal"=w430:bool)  [unwired: 1 in, 5 out]
            n199 = Unbundle By Name(w428) -> ("Peripherals.AISAS Mech.lvclass"=w429:refnum<class "AISAS Mech.lvclass">)
            n200 = call "Write AISAS check.vi"("error in (no error)"=w432, "AISAS check"=w430, "AISAS Mech in"=w429) -> ("error out"=w431:errorcluster, "AISAS Mech out"=w426:refnum<class "AISAS Mech.lvclass">)  [unwired: 7 in]
            n201 = Bundle By Name(cluster=w428, "Peripherals.AISAS Mech.lvclass"=w426) -> (w427:T15)
            n202 = Insert Into Array(array=w425, new element=Main_Program_States."Wait for Event" ("new element/subarray")) -> (w424:T18[])  [unwired: 1 in]
          }
          event "scmp nohyde": Value Change {
            n203 = event-data() -> ("NewVal"=w433:bool)  [unwired: 1 in, 5 out]
            n204 = property on="AISAS verification" class="Bool (strict)"("Visible"=w433) -> ()  [unwired: 2 in, 2 out]
            n205 = property on="Dark/Flat" class="Bool (strict)"("Visible"=w433) -> ()  [unwired: 2 in, 2 out]
            n206 = property on="Calib image" class="IntGraph (strict)"("Visible"=w433) -> ()  [unwired: 2 in, 2 out]
            n207 = property on="Processing" class="Bool (strict)"("Visible"=w433) -> ()  [unwired: 2 in, 2 out]
            n208 = property on="Run Dark" class="Bool"("Visible"=w433) -> ()  [unwired: 2 in, 2 out]
            n209 = Insert Into Array(array=w435, new element=Main_Program_States."Wait for Event" ("new element/subarray")) -> (w434:T18[])  [unwired: 1 in]
          }
          event "Print scr1": Value Change {
            n210 = event-data() -> ()  [unwired: 1 in, 6 out]
            n211 = case shown="\"Snapshots\"" "Tab Control" {
              tunnel: ["snapshot_live" "cbk_cmd" "engineering_data" "misc"] -> w439
              frame "Snapshots" {
              }
              frame "Cookbooks Commands" {
              }
              frame "Engineering Data" {
              }
              frame "Misc" {
              }
            }
            n212 = disable-structure shown="Enabled" {
              disable-tunnel: w443 -> [w455 w459]
              disable-tunnel: w442 -> [w454 w457]
              disable-tunnel: [w452 w458] -> w441
              disable-tunnel: w439 -> [_ w456]
              frame Disabled {
                n213 = invoke class="VI" method="FP.Get Image"(error in=w455) -> (error out=w453:errorcluster, "image data"=w451:T25)  [unwired: 5 in, 4 out]
                n214 = call "SCMP - print screen.vi"("error in (no error)"=w453, "image data"=w451, "FITS Header in"=w454) -> ("error out"=w452:errorcluster)  [unwired: 7 in, 1 out]
              }
              frame Enabled {
                n215 = call "SCMP - print screen RT2.vi"("error in (no error)"=w459, "Source"=w456, "FITS Header in"=w457) -> ("error out"=w458:errorcluster)  [unwired: 7 in, 1 out]
              }
            }
            n216 = Insert Into Array(array=w445, new element=Main_Program_States."Wait for Event" ("new element/subarray")) -> (w444:T18[])  [unwired: 1 in]
          }
        }
      }
      frame "Periodic Check" {
        # "funkcia AISAS auto off:\nvypnutie tlac. Motors v pripade chyby"
        # "2sec interval (po event timeout case)"
        n217 = for {
          tunnel: [w500] -> w470 mode=indexing
          tunnel: w486 -> [w498]
          tunnel: [w499] -> w490
          tunnel: w478 -> [w497] mode=indexing
          n218 = call-dynamic "Cam temp.vi"("error in (no error)"=w498, "Camera.lvclass"=w497) -> ("error out"=w499:errorcluster, "Temp"=w500:dbl)  [unwired: 8 in]
        }
        n219 = Bundle By Name(cluster=w487, "Camera Temp"=w470, "Observer"="Observer", "Comment"="Comment", "Occulter size"="Size") -> (w484:T15)
        n220 = Index Array(array=w470) -> (element #1=→"Camera 1 Temp [C}":dbl, element #2=→"Camera 2 Temp [C}":dbl)  [unwired: 2 in]
        n221 = global write "Global - pR netw comm.vi" "Pointer IP add"("Pointer IP") -> ()
        n222 = Unbundle By Name(w484) -> ("Peripherals"=w485:T17)
        n223 = call "Check.vi"("Peripherals in"=w485, "error in (no error)"=w490) -> ("error out"=w482:errorcluster, "auto off?"=w480:bool, "Peripherals out"=w483:T17, "auto off resp"=w489:string)  [unwired: 5 in, 1 out]
        n224 = Bundle By Name(cluster=w484, "Peripherals"=w483) -> (w475:T15)
        n225 = case shown="True" w480 {
          tunnel: w482 -> [w501 w502]
          tunnel: [w501 w504] -> w481
          frame False {
          }
          frame True {
            n226 = property on="Motors" class="Bool (strict)"("Val(Sgnl)"=FALSE ("Value (Signaling)")) -> (error out=w503:errorcluster)  [unwired: 2 in, 1 out]
            n227 = Merge Errors(w502, w503) -> (w504:errorcluster)
          }
        }
        n228 = case shown="Error" w481 {
          selector: w481 -> [w507 w508]
          tunnel: [w507 w512] -> w468
          tunnel: w489 -> [_ w509]
          tunnel: ["" ("Last Log Entry") w511] -> w488
          frame No Error {
          }
          frame Error {
            n229 = call "SCMP - Write log v2.vi"("Error to log"=w508, "data to end"=w509, "data"="AISAS Check ") -> ("error out"=w512:errorcluster, "Last Log Entry"=w511:string)  [unwired: 6 in, 1 out]
          }
        }
        n230 = call "Check Connection.vi"("error in (no error)"=w468) -> ("error out"=w465:errorcluster, "Connected?"=w463:bool, "Log Entry"=w466:string)  [unwired: 8 in]
        "Network\nconnected" <- w463
        n231 = case shown="False" w463 {
          tunnel: [T19."Disabled and Grayed Out" ("Disabled") T19."Enabled" ("Disabled")] -> w462
          tunnel: [T19."Enabled" ("Disabled") T19."Disabled and Grayed Out" ("Disabled")] -> w461
          frame True {
          }
          frame False {
          }
        }
        n232 = Bundle By Name(cluster=w475, "periodic check count"=0) -> (w473:T15)
        n233 = Build Array(Main_Program_States."Wait for Event" ("Next State")) -> (w471:T18[])
        n234 = Concatenate Strings(w488, w466) -> (w467:string)
        n235 = property on="Looback disable" class="Bool (strict)"(error in=w465, "DisabledEnum"=w461) -> (error out=w464:errorcluster)  [unwired: 1 in, 1 out]
        n236 = property on="Pointer IP" class="Str"("DisabledEnum"=w462) -> ()  [unwired: 2 in, 2 out]
      }
      frame "Update Image" {
        # "comp flip 180\nscd rot 180"
        n237 = call "SCMP - darkflat.vi"("error in (no error)"=w517, "Dark/Flat"="Dark/Flat", "Image Data Cluser"=w518) -> ("error out"=w516:errorcluster, "Raw Image Data2"=w525:u16[][], "Raw Image Data1"=w526:u16[][], "Y scale"=w514:i32, "Image Data"=w515:u32[][])  [unwired: 4 in]
        n238 = Unbundle By Name(w522) -> ("FITS paths"=w523:path[])
        n239 = call "Neo - Calculate Image Statistics and Histogram2.vi"("Image In"=w526) -> ("Histogram Graph"=→"Histogram Graph":T2, "Mean ADU"=→"Mean ADU":dbl)  [unwired: 8 in, 1 out]
        n240 = call "SCD - Determine Image Sharpness from 2D Derivative.vi"("Image In"=w526) -> ("Sharpness"=→"Sharpness":dbl)  [unwired: 9 in, 1 out]
        n241 = call "SCD - Determine Image Sharpness from 2D Derivative.vi"("Image In"=w525) -> ("Sharpness"=→"Sharpness 2":dbl)  [unwired: 9 in, 1 out]
        n242 = call "Neo - Calculate Image Statistics and Histogram2.vi"("Image In"=w525) -> ("Histogram Graph"=→"Histogram Graph 2":T2, "Mean ADU"=→"Mean ADU 2":dbl)  [unwired: 8 in, 1 out]
        n243 = Index Array(array=w523) -> (element #1=→"Camera FITS file path":path, element #2=→"Camera FITS file path 2":path)  [unwired: 2 in]
        n244 = disable-structure shown="SCMP==COMP, Default" {
          disable-tunnel: w515 -> [w542 w555]
          disable-tunnel: w525 -> [w545 _]
          disable-tunnel: w514 -> [w544 _]
          disable-tunnel: w516 -> [w538 w556]
          disable-tunnel: [w543 w556] -> w519
          frame condition #0 (active) {
            n245 = call "SCMP - rot180 array.vi"("pic op (noop)"=enum16{"noop", "Rot180", "Flip180"}."Flip180", "A in"=w542) -> ("A out"=w541:u32[][])  [unwired: 9 in]
            n246 = To Unsigned Word Integer(number=w541) -> (unsigned 16bit integer=→"Camera T Image Zoom" →"Camera T Image":u16[][])
            n247 = case shown="True" "Auto scale" {
              tunnel: w544 -> [_ w550]
              tunnel: [w546 w549] -> w543
              tunnel: w538 -> [w546 w547]
              frame False {
              }
              frame True {
                n248 = To Double Precision Float(number=w550) -> (double precision float=w548:dbl)
                n249 = Divide(x=w548, y=2.0) -> (x/y=w551:dbl)
                n250 = property on="Camera T Image Zoom" class="IntGraph (strict)"(error in=w547, "YScale.Maximum"=w551) -> (error out=w549:errorcluster)  [unwired: 1 in, 1 out]
              }
            }
            "Camera R Image" <- w545
          }
          frame condition #1 {
            n251 = call "SCMP - rot180 array.vi"("pic op (noop)"=enum16{"noop", "Rot180", "Flip180"}."Rot180", "A in"=w555) -> ("A out"=→"Camera Image":u32[][])  [unwired: 9 in]
          }
        }
        n252 = Unbundle By Name(w522) -> ("Time Stamp Array"=w521:timestamp[])
        n253 = Index Array(array=w521) -> (element #1=→"Timestamp":timestamp, element #2=→"Timestamp 2":timestamp)  [unwired: 2 in]
      }
      frame "Snap Images" {
        n254 = call "Snap.vi"("Save Data to FITS? (F)"="Save Data to FITS?", "error in"=w575, "FITS/UI"=w573, "Cameras in"=w574) -> ("error out"=w570:errorcluster, "FITS/UI out"=w567:T15, "Image Data Arr"=w559:u16[][][], "Cameras out"=w572:refnum<class "Camera.lvclass">[])  [unwired: 4 in]
        n255 = To Unsigned Long Integer(number=w559) -> (unsigned 32bit integer=w557:u32[][][])
        n256 = Bundle By Name(cluster=w560, "Image Data Arr"=w557) -> (w558:T21)
        n257 = call "SCMP - Write log v2.vi"("Error to log"=w570, "data"="Snap Single Image") -> ("error out"=w569:errorcluster, "Last Log Entry"=w568:string)  [unwired: 7 in, 1 out]
        n258 = Insert Into Array(array=w565, index=0, new element #1=Main_Program_States."Update Image" ("Next State"), new element #2=Main_Program_States."Wait for Event" ("new element/subarray")) -> (w564:T18[])
      }
      frame "Live Preview" {
        n259 = case shown="True" "Live Preview" {
          tunnel: w585 -> [w589 w610]
          tunnel: w584 -> [w587 w596]
          tunnel: w583 -> [w588 w608]
          tunnel: [w587 w595] -> w582
          tunnel: [w589 w609] -> w580
          tunnel: [w590 w592] -> w577
          tunnel: [w588 w602] -> w581
          tunnel: w578 -> [w590 w593]
          tunnel: [w586 w594] -> w576
          frame False {
            w586 = T18[] [enum."Wait for Event"] items=["Initialize", "Wait for Event", "Periodic Check", "Update UI", "Update Camera UI", "Load Cookbook", "Run Cookbook", "Snap Images", "Live Preview", "Set Filter Wheel", "Set Calibration Wheel", "AISAS Motors on/off", "AISAS Move", "Move AISAS Mechanisms", "Stop", "Change Camera Exposure", "Change Camera Stage Position", "Set Camera AOI", "Andor Adv Settings", "Update Image", "Run Dark", "Calib acq", "Process Calib"]
          }
          frame True {
            w594 = T18[] [enum."Update Image", enum."Wait for Event", enum."Live Preview"] items=["Initialize", "Wait for Event", "Periodic Check", "Update UI", "Update Camera UI", "Load Cookbook", "Run Cookbook", "Snap Images", "Live Preview", "Set Filter Wheel", "Set Calibration Wheel", "AISAS Motors on/off", "AISAS Move", "Move AISAS Mechanisms", "Stop", "Change Camera Exposure", "Change Camera Stage Position", "Set Camera AOI", "Andor Adv Settings", "Update Image", "Run Dark", "Calib acq", "Process Calib"]
            n260 = disable-structure shown="SCMP==COMP, Default" {
              disable-tunnel: "Wavelength [nm]" -> [w612 w613]
              disable-tunnel: [w611 w614] -> w604
              frame condition #0 (active) {
                n261 = call "CoMP-S Tune LCVR.vi"("Wavelength (nm)"=w612) -> ("Required LCVR Voltages"=w611:dbl[])  [unwired: 9 in, 1 out]
              }
              frame condition #1 {
                n262 = call "SCD - Use Global Variables to Compute LCVR Voltages.vi"("Wavelength (nm)"=w613) -> ("Required LCVR Voltages"=w614:dbl[])  [unwired: 1 in, 1 out]
              }
            }
            n263 = Bundle By Name(cluster=w608, "Tuning Voltages"=w604, "Wavelength (nm)"="Wavelength [nm]") -> (w605:T15)
            n264 = local read "Save Data to FITS?"() -> (w599:bool)
            n265 = Build Array(w604) -> (w603:dbl[][])
            n266 = Build Array(w605) -> (w606:T15[])
            n267 = call "Data Acquisition - v8.vi"("Cameras in"=w596, "Save to FITS?"=w599, "error in"=w610, "LCVR Voltages"=w603, "Headers In"=w606) -> ("Cameras out"=w595:refnum<class "Camera.lvclass">[], "Image data"=w601:u32[][], "Image data2"=w600:u32[][], "Headers Out"=w598:T15[], "error out"=w609:errorcluster)  [unwired: 5 in, 1 out]
            n268 = Index Array(array=w598, index=0) -> (element=w602:T15)
            n269 = Build Array(w601, w600) -> (w591:u32[][][])
            n270 = Bundle By Name(cluster=w593, "Image Data Arr"=w591) -> (w592:T21)
          }
        }
      }
      frame "Load Cookbook" {
        n271 = Unbundle By Name(w617) -> ("load preset cbk"=w625:bool)
        n272 = Unbundle By Name(w617) -> ("Cameras"=w616:T12)
        n273 = control-ref of="preset cbk"() -> (w615:refnum<vi>)
        n274 = call "SCMP - Read Cookbook.vi"("error in"=w640, "load preset cbk?"=w625, "preset cbk ring ref"=w615) -> ("error out"=w622:errorcluster, "Recipe Files"=→"Recipe Files":string[], "# of Recipes"=w642:i16, "Cookbook"=→"Cookbook":T13, "min Cookbook Exposure [s]"=w636:dbl, "Selected Cookbook"=w637:path, "Cookbook Comments"=→"Cookbook Comments":string)  [unwired: 2 in]
        "Selected Cookbook" <- w637
        "min Cookbook Exposure [s]" <- w636
        n275 = call "Cams select.vi"("Cameras"=w616, "Cameras in"=w620) -> ("Cams selection"=w619:refnum<class "Camera.lvclass">[])  [unwired: 8 in, 1 out]
        n276 = Index Array(array=w619) -> (element=w618:refnum<class "Camera.lvclass">)  [unwired: 1 in]
        n277 = Greater Than 0?(x=w636) -> (x > 0?=w635:bool)
        n278 = case shown="True" w635 {
          tunnel: w636 -> [_ w653]
          tunnel: w622 -> [w650 w656]
          tunnel: [w650 w655] -> w621
          tunnel: w618 -> [_ w654]
          frame False {
          }
          frame True {
            n279 = call-dynamic "Check FPS.vi"("Set Exp or Check Fps (Set Exp)"=enum16{"Set Exp", "Check FPS"}."Check FPS", "error in (no error)"=w656, "Exposure [s]"=w653, "Camera in"=w654) -> ("error out"=w655:errorcluster, "FPS"=w651:dbl)  [unwired: 5 in, 1 out]
            n280 = local write "max Cookbook FPS"(w651) -> ()
          }
        }
        n281 = Unbundle By Name(w621) -> ("status"=w626:bool)
        n282 = case shown="No Error" w621 {
          selector: w621 -> [w659 w666]
          tunnel: w642 -> [w665 _]
          tunnel: w637 -> [w663 w671]
          tunnel: [w664 w669] -> w649
          tunnel: [w658 w666] -> w645
          frame No Error {
            n283 = Strip Path(path=w663) -> (name=w661:string)  [unwired: 1 out]
            "cbk name" <- w661
            n284 = property on="Run Cookbook" class="Bool"(error in=w659, "DisabledEnum"=T19."Enabled" ("Disabled")) -> (error out=w658:errorcluster)  [unwired: 1 in, 1 out]
            n285 = Concatenate Strings("Loaded Cookbook" ("data"), "\t", w661) -> (w664:string)
            "# of Recipes" <- w665
          }
          frame Error {
            n286 = Strip Path(path=w671) -> (name=w670:string)  [unwired: 1 out]
            n287 = property on="Run Cookbook" class="Bool"("DisabledEnum"=T19."Disabled and Grayed Out" ("Disabled")) -> ()  [unwired: 2 in, 2 out]
            n288 = Concatenate Strings("Error Loading Cookbook" ("data"), "\t", w670) -> (w669:string)
          }
        }
        n289 = Not(x=w626) -> (.not. x?=w623:bool)
        n290 = And(x=w623, y=w625) -> (x .and. y?=w624:bool)
        n291 = Strip Path(path=w637) -> (name=w646:string)  [unwired: 1 out]
        n292 = Select(t=Main_Program_States."Run Cookbook", s=w624, f=Main_Program_States."Wait for Event" ("Next State")) -> (s? t:f=w627:T18)
        n293 = Bundle By Name(cluster=w617, "Cookbook"=w646, "load preset cbk"=FALSE) -> (w647:T15)
        n294 = call "SCMP - Write log v2.vi"("Error to log"=w645, "data"=w649) -> ("error out"=w639:errorcluster, "Last Log Entry"=w648:string)  [unwired: 7 in, 1 out]
        n295 = Insert Into Array(array=w633, index=0, new element=w627) -> (w632:T18[])
        n296 = call <vilib>:"Clear Errors.vi"("error in (no error)"=w639) -> ("error out"=w638:errorcluster)  [unwired: 5 in, 1 out]
      }
      frame "Run Cookbook" {
        # "skusam delay kvoli lv crash\npo pre-setup"
        # "beep na konci ak cbk trval dlhsie ako 60 sec"
        n297 = local read "cbk name"() -> (w698:string)
        n298 = property on="Looback disable" class="Bool (strict)"(error in=w679) -> (error out=w678:errorcluster, "DisabledEnum"=w677:T19)  [unwired: 1 in, 1 out]
        n299 = Concatenate Strings("Run Cookbook" ("data"), "\t", w698) -> (w702:string)
        n300 = Equal?(x=w677, y=T19."Enabled") -> (x = y?=w673:bool)
        n301 = call "SCMP - Write log v2.vi"("Error to log"=w678, "data"=w702) -> ("error out"=w701:errorcluster, "Last Log Entry"=w695:string)  [unwired: 7 in, 1 out]
        n302 = And(x=w673, y="Looback disable") -> (x .and. y?=w674:bool)
        n303 = flat-sequence {
          tunnel: [w723] -> w711
          tunnel: w701 -> [w723]
          tunnel: [w722] -> w708
          frame #0 {
            n304 = Get Date/Time In Seconds() -> (seconds since 1Jan1904=w722:timestamp)
          }
        }
        n305 = local read "Lyot Filter Temp [C]"() -> (w680:dbl)
        n306 = local read "Motors"() -> (w713:bool)
        n307 = local read "Cookbook"() -> (w716:T13)
        n308 = call "Run Cookbook.vi"("Cookbook"=w716, "Mod/Seq"="Mod/Seq", "Disable pR"=w674, "Save to FITS?"="Save Data to FITS?", "limit max FPS to:"="limit max Cookbook FPS to:", "Motors"=w713, "Lyot Filter Temp [C]"=w680, "Error in"=w711, "Cameras in"=w693, "FITS Header In"=w714) -> ("Result"=w707:string, "FITS Path Out"=→"FITS Path from Last Recipe Acquiring Data":path, "Cameras out"=w692:refnum<class "Camera.lvclass">[], "Updated Header"=w703:T15, "Error out"=w710:errorcluster)  [unwired: 1 in]
        n309 = flat-sequence {
          tunnel: [w721] -> w687
          tunnel: w710 -> [w721]
          tunnel: [w720] -> w709
          frame #0 {
            n310 = Get Date/Time In Seconds() -> (seconds since 1Jan1904=w720:timestamp)
          }
        }
        n311 = Subtract(x=w709, y=w708) -> (x-y=w686:dbl)
        n312 = Greater Or Equal?(x=w686, y=60.0) -> (x >= y?=w684:bool)
        n313 = Format Date/Time String(time format string (%c)="%M:%S] ", seconds (now)=w686) -> (date/time string=w705:string)  [unwired: 1 in]
        n314 = case shown="True" w684 {
          frame False {
          }
          frame True {
            n315 = call "SCMP - Cbk end sound.vi"() -> ()  [unwired: 12 in]
          }
        }
        n316 = Concatenate Strings(w707, " [" ("string"), w705) -> (w719:string)
        n317 = call "SCMP - Write log v2.vi"("Error to log"=w687, "data"=w719) -> ("error out"=w682:errorcluster, "Last Log Entry"=w696:string)  [unwired: 7 in, 1 out]
        n318 = Concatenate Strings(w696, w695) -> (w697:string)
        n319 = Insert Into Array(array=w691, index=0, new element=Main_Program_States."Update UI" ("Beginning State")) -> (w690:T18[])
        n320 = call "Time Delay"("error in (no error)"=w682, "Delay Time (s)"=1.0) -> ("error out"=w681:errorcluster)  [unwired: 9 in]
      }
      frame "Set Filter Wheel" {
        n321 = disable-structure shown="SCMP==COMP, Default" {
          disable-tunnel: w737 -> [w748 w754]
          disable-tunnel: [w747 w753] -> w736
          disable-tunnel: [w741 w749] -> w734
          disable-tunnel: [w745 w752] -> w730
          disable-tunnel: w731 -> [w746 w751]
          frame condition #0 {
            n322 = disable-structure shown="Disabled" {
              frame Disabled {
                # "old filter wheel vi"
                n323 = call "Optec IFW3 - Standalone.vi"() -> ()  [unwired: 11 in, 1 out]
              }
              frame Enabled {
              }
            }
            n324 = call "SCD - wavelenght.vi"("SCD Emission Line Filter"="Emission Line Filters") -> ("Numeric"=w742:dbl)  [unwired: 10 in]
            n325 = call "Optec IFW3 - Set Position with Error Handling.vi"("error in"=w748, "Emission Line Filter"="Emission Line Filters", "Filter Wheel Selector"=T24."Emission Line Filters") -> ("error out"=w741:errorcluster, "Actual Position (1-9)"=w747:i32)  [unwired: 6 in, 1 out]
            n326 = Bundle By Name(cluster=w746, "SCD Emission Line Filter"="Emission Line Filters", "Wavelength (nm)"=w742) -> (w745:T15)
          }
          frame condition #1 (active) {
            n327 = call "CoMP-S Mechanism - FW.vi"("error in (no error)"=w754, "Emission Line Filters [530.3 nm]"="Andover Filter Wheel", "Filter Wheel Selector"=T24."Emission Line Filters") -> ("error out"=w749:errorcluster, "Position"=w753:i32)  [unwired: 5 in, 2 out]
            n328 = Bundle By Name(cluster=w751, "COMP-S Andover Filter Wheel"="Andover Filter Wheel") -> (w752:T15)
          }
        }
        n329 = Number To Decimal String(number=w736) -> (decimal integer string=w732:string)  [unwired: 1 in]
        n330 = Concatenate Strings("Filter Wheel position:" ("data"), "\t", w732) -> (w733:string)
        n331 = call "SCMP - Write log v2.vi"("Error to log"=w734, "data"=w733) -> ("error out"=w735:errorcluster, "Last Log Entry"=w739:string)  [unwired: 7 in, 1 out]
        n332 = Insert Into Array(array=w727, index=0, new element=Main_Program_States."Update UI" ("Next State")) -> (w726:T18[])
      }
      frame "Set Calibration Wheel" {
        n333 = disable-structure shown="SCMP==COMP, Default" {
          disable-tunnel: w766 -> [w773 w781]
          disable-tunnel: [w778 w783] -> w764
          disable-tunnel: [w777 w782] -> w762
          disable-tunnel: [w775 w779] -> w760
          disable-tunnel: w761 -> [w776 w779]
          frame condition #0 {
            n334 = disable-structure shown="Disabled" {
              frame Disabled {
                # "old filter wheel vi"
                n335 = call "Optec IFW3 - Standalone.vi"() -> ()  [unwired: 11 in, 1 out]
              }
              frame Enabled {
              }
            }
            n336 = Bundle By Name(cluster=w776, "SCD Calibration Optics"="Calibration Optics") -> (w775:T15)
            n337 = call "Optec IFW3 - Set Position with Error Handling.vi"("error in"=w773, "SCD Calibration Optics"="Calibration Optics", "Filter Wheel Selector"=T24."Calibration Polarizers") -> ("error out"=w778:errorcluster, "Actual Position (1-9)"=w777:i32)  [unwired: 6 in, 1 out]
          }
          frame condition #1 (active) {
            n338 = Unbundle By Name(w779) -> ("COMP-S Calibration Wheel"=w780:T7)
            n339 = call "CoMP-S Mechanism - FW.vi"("error in (no error)"=w781, "Calibration Polarizer Filters [Dark]"=w780, "Filter Wheel Selector"=T24."Calibration Polarizers") -> ("error out"=w783:errorcluster, "Position"=w782:i32)  [unwired: 5 in, 2 out]
          }
        }
        n340 = Number To Decimal String(number=w762) -> (decimal integer string=w770:string)  [unwired: 1 in]
        n341 = Concatenate Strings("Calibration Wheel position:" ("data"), "\t", w770) -> (w763:string)
        n342 = call "SCMP - Write log v2.vi"("Error to log"=w764, "data"=w763) -> ("error out"=w765:errorcluster, "Last Log Entry"=w768:string)  [unwired: 7 in, 1 out]
        n343 = Insert Into Array(array=w758, new element=Main_Program_States."Wait for Event" ("Next State")) -> (w757:T18[])  [unwired: 1 in]
      }
      frame "AISAS Motors on/off" {
        n344 = Unbundle By Name(w792) -> ("Peripherals"=w794:T17)
        n345 = Select(t="on" ("data"), s="Motors", f="off" ("data")) -> (s? t:f=w799:string)
        n346 = call "Mech on_off.vi"("Peripherals in"=w794, "error in (no error)"=w797, "Motors"="Motors") -> ("error out"=w804:errorcluster, "auto off log"=w790:string, "Peripherals out"=w793:T17)  [unwired: 6 in]
        n347 = Bundle By Name(cluster=w792, "Peripherals"=w793) -> (w791:T15)
        n348 = Concatenate Strings("AISAS Motors " ("data"), w799, w790) -> (w798:string)
        n349 = call "SCMP - Write log v2.vi"("Error to log"=w804, "data"=w798) -> ("error out"=w796:errorcluster, "Last Log Entry"=w795:string)  [unwired: 7 in, 1 out]
        n350 = Insert Into Array(array=w788, index=0, new element=Main_Program_States."Wait for Event" ("Next State")) -> (w787:T18[])
      }
      frame "AISAS Move" {
        n351 = Unbundle By Name(w827) -> ("Peripherals.AISAS Mech.lvclass"=w825:refnum<class "AISAS Mech.lvclass">)
        n352 = call "Move.vi"("error in (no error)"=w826, "AISAS Mech in"=w825) -> ("error out"=w824:errorcluster, "AISAS Mech out"=w822:refnum<class "AISAS Mech.lvclass">)  [unwired: 7 in, 1 out]
        n353 = Bundle By Name(cluster=w827, "Peripherals.AISAS Mech.lvclass"=w822) -> (w816:T15)
        n354 = call "Read value.vi"("error in (no error)"=w824, "AISAS Mech in"=w822) -> ("error out"=w823:errorcluster, "Rotation"=w815:T11, "Focus"=w814:T5, "Diffuser"=w818:T10, "Motor"=w817:T23, "Value (String)"=w819:string, "Motor (String)"=w821:string)  [unwired: 3 in]
        n355 = Concatenate Strings("AISAS " ("data"), w821, " set to: " ("data"), w819) -> (w829:string)
        n356 = call "SCMP - Write log v2.vi"("Error to log"=w823, "data"=w829) -> ("error out"=w813:errorcluster, "Last Log Entry"=w828:string)  [unwired: 7 in, 1 out]
        n357 = case shown="\"Diffuser \"" w817 {
          tunnel: w818 -> [w833 _ _]
          tunnel: w816 -> [w834 w837 w840]
          tunnel: w814 -> [_ w836 _]
          tunnel: w815 -> [_ _ w839]
          tunnel: [w832 w835 w838] -> w811
          frame "Diffuser " {
            n358 = Bundle By Name(cluster=w834, "Light Shapping Diffuser"=w833) -> (w832:T15)
          }
          frame "Focus" {
            n359 = Bundle By Name(cluster=w837, "Objective Lens Position (mm)"=w836) -> (w835:T15)
          }
          frame "Rotation" {
            n360 = Bundle By Name(cluster=w840, "FOV Rotation (deg)"=w839) -> (w838:T15)
          }
        }
        n361 = call "SCMP write init xml.vi"("error in (no error)"=w813, "FITS Header In"=w811) -> ("error out"=w812:errorcluster)  [unwired: 8 in, 1 out]
        n362 = Insert Into Array(array=w809, index=0, new element=Main_Program_States."Update UI" ("Next State")) -> (w808:T18[])
      }
      frame "Change Camera Stage Position" {
        n363 = Build Array("PI cam1 (mm)", "PI cam2 (mm)", "PI cam3 (mm)") -> (w853:T3[])
        n364 = call "SCMP - Control PI Stage Position2.vi"("error in"=w858, "Absolute (F) or \nRelative (T) Move"=FALSE ("Absolute (F) or \nRelative (T) Move"), "set values"=w853) -> ("error out"=w854:errorcluster, "PI set?"=w850:bool, "Position"=w851:dbl[])  [unwired: 6 in]
        n365 = case shown="True" w850 {
          tunnel: ["" w874] -> w859
          tunnel: w849 -> [w861 w873]
          tunnel: [w861 w872] -> w856
          tunnel: [w862 w871] -> w855
          tunnel: w854 -> [w862 w864]
          tunnel: w851 -> [_ w863]
          frame False {
          }
          frame True {
            n366 = Bundle By Name(cluster=w873, "Camera PI (mm)"=w863) -> (w872:T15)
            n367 = Number To Fractional String(number=w863, width (-)=i16 6, precision (6)=i16 2) -> (F-format string=w869:string[])  [unwired: 1 in]
            n368 = Concatenate Strings("Camera PI:" ("Recent Log"), w869, "\n" ("string")) -> (w868:string)
            n369 = call "SCMP - Write log v2.vi"("Error to log"=w864, "data"=w868) -> ("error out"=w871:errorcluster, "Last Log Entry"=w874:string)  [unwired: 7 in, 1 out]
          }
        }
        n370 = Insert Into Array(array=w844, index=0, new element=Main_Program_States."Update UI" ("Next State")) -> (w843:T18[])
      }
      frame "Change Camera Exposure" {
        n371 = Unbundle By Name(w889) -> ("Cameras"=w891:T12)
        n372 = call "Cams select.vi"("Cameras"=w891, "Cameras in"=w885) -> ("Cams selection"=w890:refnum<class "Camera.lvclass">[], "Cams indx"=w887:i32)  [unwired: 8 in]
        n373 = for {
          shift-right: [w899] -> w880
          shift-left: w894 -> [w901]
          tunnel: [w897] -> w883
          tunnel: w890 -> [w900] mode=indexing
          tunnel: "Exposure (s)" -> [w898]
          tunnel: [w896] -> w886 mode=indexing
          n374 = call-dynamic "Set exp.vi"("error in (no error)"=w901, "Exposure (s)"=w898, "Camera in"=w900) -> ("error out"=w899:errorcluster, "Exposure (s) out"=w897:dbl, "Camera out"=w896:refnum<class "Camera.lvclass">)  [unwired: 6 in]
        }
        n375 = Replace Array Subset(array=w885, new element=w886, index=w887) -> (w884:refnum<class "Camera.lvclass">[])
        n376 = Format Into String(format string="Camera Exposure: %.2ps " ("data"), error in=w880, w883) -> (resulting string=w881:string, error out=w879:errorcluster)  [unwired: 1 in]
        n377 = call "SCMP - Write log v2.vi"("Error to log"=w879, "data"=w881) -> ("error out"=w893:errorcluster, "Last Log Entry"=w895:string)  [unwired: 7 in, 1 out]
        n378 = Insert Into Array(array=w878, index=0, new element=Main_Program_States."Update UI" ("Beginning State")) -> (w877:T18[])
      }
      frame "Set Camera AOI" {
        n379 = Unbundle By Name(w906) -> ("Cameras"=w915:T12)
        n380 = call "Cams select.vi"("Cameras"=w915, "Cameras in"=w913) -> ("Cams selection"=w909:refnum<class "Camera.lvclass">[], "Cams indx"=w914:i32)  [unwired: 8 in]
        n381 = for {
          shift-right: [w925] -> w911
          shift-left: w912 -> [w926]
          tunnel: w909 -> [w924] mode=indexing
          tunnel: [w923] -> w908 mode=indexing
          tunnel: "Binning" -> [w922]
          n382 = call-dynamic "Set binning.vi"("error in (no error)"=w926, "Binning"=w922, "Camera in"=w924) -> ("error out"=w925:errorcluster, "Camera out"=w923:refnum<class "Camera.lvclass">)  [unwired: 7 in]
        }
        n383 = Replace Array Subset(array=w913, new element=w908, index=w914) -> (w910:refnum<class "Camera.lvclass">[])
        n384 = property on="Binning" class="Enum (strict)"() -> ("RingText.Text"=w917:string)  [unwired: 2 in, 2 out]
        n385 = Concatenate Strings("Camera Binning: " ("Recent Log"), w917) -> (w920:string)
        n386 = call "SCMP - Write log v2.vi"("Error to log"=w911, "data"=w920) -> ("error out"=w918:errorcluster, "Last Log Entry"=w919:string)  [unwired: 7 in, 1 out]
        n387 = Insert Into Array(array=w905, index=0, new element=Main_Program_States."Update UI" ("Beginning State")) -> (w904:T18[])
      }
      frame "Andor Adv Settings" {
        n388 = call "Cams select.vi"("Cameras"=Cameras_select."Andor", "Cameras in"=w935) -> ("Cams selection"=w938:refnum<class "Camera.lvclass">[], "Cams indx"=w936:i32)  [unwired: 8 in]
        n389 = for {
          tunnel: w938 -> [w956] mode=indexing
          tunnel: [w955] -> w942 mode=indexing
          n390 = call-dynamic "Read Cam info.vi"("Camera in"=w956) -> ("Handle"=w955:i32)  [unwired: 5 in, 9 out]
        }
        n391 = Index Array(array=w942) -> (element #1=w941:i32, element #2=w940:i32)  [unwired: 2 in]
        n392 = call-by-ref "SCMP Andor setupdialog.vi"(error in=w946, "Handle 2"=w940, "Handle"=w941) -> (error out=w929:errorcluster, "scmp nohyde out"=w927:bool)  [unwired: 10 in, 1 out]
        n393 = property on="scmp nohyde" class="Bool (strict)"(error in=w929, "Val(Sgnl)"=w927) -> (error out=w928:errorcluster)  [unwired: 1 in, 1 out]
        n394 = for {
          tunnel: w938 -> [w954] mode=indexing
          shift-right: [w950] -> w939
          shift-left: w928 -> [w951]
          tunnel: [w947] -> w937 mode=indexing
          n395 = To More Specific Class(target class=refnum<class "Andor.lvclass"> refnum ("Andor.lvclass"), reference=w954) -> (specific class reference=w953:refnum<class "Andor.lvclass">)  [unwired: 1 in, 1 out]
          n396 = call "Andor Neo check.vi"("error in"=w951, "Andor.lvclass"=w953) -> ("error out"=w950:errorcluster, "Andor.lvclass out"=w949:refnum<class "Andor.lvclass">)  [unwired: 5 in, 3 out]
          n397 = To More Generic Class(target class=refnum<class "Camera.lvclass"> refnum ("Camera.lvclass"), reference=w949) -> (generic class reference=w947:refnum<class "Camera.lvclass">)
        }
        n398 = Replace Array Subset(array=w935, new element=w937, index=w936) -> (w934:refnum<class "Camera.lvclass">[])
        n399 = Insert Into Array(array=w932, index=0, new element=Main_Program_States."Update UI" ("Beginning State")) -> (w931:T18[])
      }
      frame "Run Dark" {
        w960 = T18[] [enum."Set Calibration Wheel", enum."Calib acq", enum."Process Calib"] items=["Initialize", "Wait for Event", "Periodic Check", "Update UI", "Update Camera UI", "Load Cookbook", "Run Cookbook", "Snap Images", "Live Preview", "Set Filter Wheel", "Set Calibration Wheel", "AISAS Motors on/off", "AISAS Move", "Move AISAS Mechanisms", "Stop", "Change Camera Exposure", "Change Camera Stage Position", "Set Camera AOI", "Andor Adv Settings", "Update Image", "Run Dark", "Calib acq", "Process Calib"]
        # "zapametanie si povodnej hodnoty fw"
        n400 = Unbundle By Name(w965) -> ("COMP-S Calibration Wheel"=w964:T7)
        n401 = Bundle By Name(cluster=w965, "Calib"=enum16{"Dark", "Flat"}."Dark", "COMP-S Calibration Wheel"=Polarization_Optics_Filter_Wheel."Dark", "COMP-S Calibration Wheel 2"=w964) -> (w963:T15)
        n402 = property on="Processing" class="Bool (strict)"(error in=w959, "Blinking"=TRUE) -> (error out=w958:errorcluster)  [unwired: 1 in, 1 out]
      }
      frame "Calib acq" {
        w968 = FALSE ("Processing")
        w971 = TRUE ("Processing")
        w977 = FALSE  # Mod/Seq
        w979 = u16 16  # Cycles
        w983 = FALSE  # Save to FITS?
        n403 = Unbundle By Name(w981) -> ("Wavelength (nm)"=w980:dbl)
        n404 = property on="Processing" class="Bool (strict)"(error in=w973, "Value"=w971, "Blinking"=w971) -> (error out=w972:errorcluster)  [unwired: 1 in, 1 out]
        n405 = disable-structure shown="SCMP==COMP, Default" {
          disable-tunnel: w980 -> [w995 w996]
          disable-tunnel: [w994 w997] -> w987
          frame condition #0 (active) {
            n406 = call "CoMP-S Tune LCVR.vi"("Wavelength (nm)"=w995) -> ("Required LCVR Voltages"=w994:dbl[])  [unwired: 9 in, 1 out]
          }
          frame condition #1 {
            n407 = call "SCD - Use Global Variables to Compute LCVR Voltages.vi"("Wavelength (nm)"=w996) -> ("Required LCVR Voltages"=w997:dbl[])  [unwired: 1 in, 1 out]
          }
        }
        n408 = local read "limit max Cookbook FPS to:"() -> (w978:dbl)
        n409 = Bundle By Name(cluster=w981, "Tuning Voltages"=w987) -> (w988:T15)
        n410 = Build Array(w987) -> (w986:dbl[][])
        n411 = Build Array(w988) -> (w989:T15[])
        n412 = call "Data Acquisition - v8.vi"("Cameras in"=w993, "Save to FITS?"=w983, "Mod/Seq"=w977, "Cycles"=w979, "Max FPS limit"=w978, "error in"=w972, "LCVR Voltages"=w986, "Headers In"=w989) -> ("Cameras out"=w992:refnum<class "Camera.lvclass">[], "Calib data"=w974:u32[][], "Headers Out"=w985:T15[], "error out"=w970:errorcluster)  [unwired: 2 in, 2 out]
        "Calib image" <- w974
        n413 = Index Array(array=w985, index=0) -> (element=w976:T15)
        n414 = Build Array(w974) -> (w975:u32[][][])
        n415 = Bundle By Name(cluster=w991, "Image Data Arr"=w975) -> (w990:T21)
        n416 = property on="Processing" class="Bool (strict)"(error in=w970, "Value"=w968, "Blinking"=w968) -> (error out=w969:errorcluster)  [unwired: 1 in, 1 out]
      }
      frame "Process Calib" {
        n417 = Unbundle By Name(w1002) -> ("Calib"=w1001:enum16{"Dark", "Flat"})
        n418 = case shown="\"Dark\", Default" w1001 {
          tunnel: w1002 -> [w1016 w1018]
          tunnel: [w1014 w1018] -> w1006
          tunnel: [w1013 w1017] -> w1005
          tunnel: w1004 -> [w1012 w1020]
          tunnel: [w1011 w1020] -> w1003
          tunnel: w1000 -> [w1008 w1019]
          tunnel: [w1008 w1019] -> w999
          tunnel: w998 -> [_ w1017]
          frame "Dark", Default {
            w1013 = T18[] [enum."Set Calibration Wheel", enum."Update Image", enum."Wait for Event"] items=["Initialize", "Wait for Event", "Periodic Check", "Update UI", "Update Camera UI", "Load Cookbook", "Run Cookbook", "Snap Images", "Live Preview", "Set Filter Wheel", "Set Calibration Wheel", "AISAS Motors on/off", "AISAS Move", "Move AISAS Mechanisms", "Stop", "Change Camera Exposure", "Change Camera Stage Position", "Set Camera AOI", "Andor Adv Settings", "Update Image", "Run Dark", "Calib acq", "Process Calib"]
            # "nastavi sa spet povodna hodnota fw"
            n419 = Unbundle By Name(w1016) -> ("COMP-S Calibration Wheel 2"=w1015:T7)
            n420 = Unbundle By Name(w1012) -> ("Image Data Arr"=w1010:u32[][][])
            n421 = Index Array(array=w1010) -> (element=w1009:u32[][])  [unwired: 3 in]
            n422 = Bundle By Name(cluster=w1016, "COMP-S Calibration Wheel"=w1015) -> (w1014:T15)
            n423 = Bundle By Name(cluster=w1012, "Dark"=w1009) -> (w1011:T21)
          }
          frame "Flat" {
          }
        }
      }
      frame "Stop" {
        w1021 = FALSE ("All Loop Stop")
        n424 = Unbundle By Name(w1023) -> ("Peripherals.PI Stages"=w1031:bool)
        n425 = call "SCMP write init xml.vi"("error in (no error)"=w1025, "FITS Header In"=w1023) -> ("error out"=w1024:errorcluster)  [unwired: 8 in, 1 out]
        n426 = global read "Global demo.vi" "demo"() -> (w1034:bool)
        n427 = Not(x=w1034) -> (.not. x?=w1032:bool)
        n428 = Compound Arithmetic op=AND(w1032, w1029, w1031) -> (w1033:bool)
        n429 = case shown="True" w1033 {
          tunnel: [FALSE w1042] -> w1035
          frame False {
          }
          frame True {
            n430 = Two Button Dialog(message="Set PI stages to parking position?", 1:"No" ("F button name (\"Cancel\")"), 2:"Yes" ("T button name (\"OK\")")) -> (T button?=w1042:bool)
          }
        }
        n431 = local write "Network\nconnected"(w1021) -> ()
        n432 = local write "Pointer ON"(w1021) -> ()
        n433 = case shown="True" w1035 {
          tunnel: w1024 -> [w1047 w1056]
          tunnel: [w1047 w1055] -> w1037
          tunnel: ["Main Loop Terminated" ("data") w1052] -> w1036
          frame False {
          }
          frame True {
            w1053 = "\n" ("string")
            n434 = disable-structure shown="SCMP==COMP, Default" {
              disable-tunnel: [w1063 w1064] -> w1057
              frame condition #0 (active) {
                n435 = global read "Globals.vi" "comp parking pos"() -> (w1063:dbl[])
              }
              frame condition #1 {
                n436 = global read "Globals.vi" "scd parking pos"() -> (w1064:dbl[])
              }
            }
            n437 = call "SCMP - Control PI Stage Position2.vi"("error in"=w1056, "Absolute (F) or \nRelative (T) Move"=FALSE ("Absolute (F) or \nRelative (T) Move"), "set values"=w1057) -> ("error out"=w1055:errorcluster, "Position"=w1051:dbl[])  [unwired: 6 in, 1 out]
            n438 = Index Array(array=w1051) -> (element #1=w1048:dbl, element #2=w1049:dbl, element #3=w1050:dbl)  [unwired: 3 in]
            n439 = Number To Fractional String(number=w1051, width (-)=i16 6, precision (6)=i16 2) -> (F-format string=w1061:string[])  [unwired: 1 in]
            n440 = local write "PI cam1 (mm)"(w1048) -> ()
            n441 = local write "PI cam2 (mm)"(w1049) -> ()
            n442 = local write "PI cam3 (mm)"(w1050) -> ()
            n443 = Concatenate Strings("Camera Moved to Positon:" ("Recent Log"), w1061, w1053, "Main Loop Terminated" ("data"), w1053) -> (w1052:string)
          }
        }
        n444 = global write "Global - All Loop Stop.vi" "All Loop Stop"(TRUE ("All Loop Stop")) -> ()
        n445 = call "SCMP - Write log v2.vi"("Error to log"=w1037, "data"=w1036) -> ("error out"=w1038:errorcluster, "Last Log Entry"=w1040:string)  [unwired: 7 in, 1 out]
        n446 = Build Array(Main_Program_States."Stop" ("Next State")) -> (w1026:T18[])
      }
    }
    "FITS Header" <- w109
    n447 = Not(x=w100) -> (.not. x?=→"Main Loop":bool)
    n448 = global read "Global - pR netw comm.vi" "Pointer ON"() -> (→"Pointer ON":bool)
    n449 = Concatenate Strings(w116, w117) -> (w115:string)
    "Latest Actions" <- w115
    n450 = local write "Main Loop Error"(w111) -> ()
    n451 = call <vilib>:"General Error Handler.vi"("error in (no error)"=w111) -> ("error out"=w112:errorcluster)  [unwired: 10 in, 4 out]
    n452 = call <vilib>:"Clear Errors.vi"("error in (no error)"=w112) -> ("error out"=w114:errorcluster)  [unwired: 5 in, 1 out]
  }
  n453 = while {
    shift-right: [w1071] -> _
    shift-left: w6 -> [w1068]
    tunnel: [FALSE ("Main Loop")] -> w39
    shift-right: [w1075] -> _
    shift-left: w38 -> [w1073]
    shift-right: [w1069] -> w27
    shift-left: w28 -> [w1072]
    stop <- w1066 stop-if-true
    # "Eng Data monitoring loop"
    n454 = call "Elapsed Time"("Time Target (s)"=w1073, "error in (no error)"=w1068) -> ("Time has Elapsed"=w1076:bool, "error out"=w1067:errorcluster)  [unwired: 10 in, 6 out]
    n455 = case shown="True" w1076 {
      tunnel: w1067 -> [w1078 w1084]
      tunnel: [w1078 w1083] -> w1070
      tunnel: w1073 -> [w1079 _]
      tunnel: [w1079 w1082] -> w1075
      tunnel: w1072 -> [w1077 w1081]
      tunnel: [w1077 w1080] -> w1069
      frame False {
      }
      frame True {
        w1082 = 10.0  # Log cadence time [s]
        # "bliknutie indikatora log loop"
        n456 = stacked-sequence {
          frame #0 {
            n457 = local write "Log Loop"(FALSE ("Log Loop")) -> ()
            n458 = Wait (ms)(milliseconds to wait=u32 200) -> ()  [unwired: 1 out]
          }
          frame #1 {
            n459 = local write "Log Loop"(TRUE ("Log Loop")) -> ()
          }
        }
        n460 = case shown="True" "Enable Data Logging" {
          tunnel: w1084 -> [w1090 w1102]
          tunnel: [w1090 w1097] -> w1083
          tunnel: w1081 -> [w1089 w1093]
          tunnel: [w1089 w1099] -> w1080
          frame False {
          }
          frame True {
            n461 = call "Read Zone Temps v2.vi"("Peripherals"=w1093, "error in"=w1102) -> ("error out"=w1092:errorcluster, "Air Temp [C]"=w1091:dbl, "Camera Body [C]"=w1103:sgl, "Pre-Filter Temp [C}"=w1100:sgl, "Peripherals out"=w1098:T17)  [unwired: 5 in]
            "Air around Camera [C]" <- w1103
            "Air around \nprefilter wheel [C]" <- w1100
            "Air around Lyot Filter [C]" <- w1091
            n462 = call "ILX Status.vi"("Peripherals in"=w1098, "error in"=w1092) -> ("error out"=w1101:errorcluster, "Temperature"=w1104:dbl, "Peripherals out"=w1099:T17)  [unwired: 4 in, 3 out]
            "Lyot Filter Temp [C]" <- w1104
            n463 = local read "Camera 1 Temp [C}"() -> (w1096:dbl)
            n464 = Build Array(w1104, w1100, w1103, w1091, w1096) -> (w1095:dbl[])
            n465 = disable-structure shown="SCMP==COMP, Default" {
              disable-tunnel: w1095 -> [w1106 w1108]
              disable-tunnel: [w1105 w1108] -> w1094
              frame condition #0 (active) {
                n466 = local read "Camera 2 Temp [C}"() -> (w1107:dbl)
                n467 = Build Array (concatenate)(w1106, w1107) -> (w1105:dbl[])
              }
              frame condition #1 {
              }
            }
            n468 = call "SCMP - Write Eng Data v2.vi"("error in"=w1101, "Temp Data"=w1094) -> ("error out"=w1097:errorcluster)  [unwired: 6 in, 3 out]
            "Eng Data Error" <- w1097
          }
        }
      }
    }
    n469 = global read "Global - All Loop Stop.vi" "All Loop Stop"() -> (w1066:bool)
    n470 = Wait (ms)(milliseconds to wait=u32 100) -> ()  [unwired: 1 out]
    n471 = call <vilib>:"Clear Errors.vi"("error in (no error)"=w1070) -> ("error out"=w1071:errorcluster)  [unwired: 5 in, 1 out]
  }
  "Log Loop" <- w39
  n472 = Unbundle By Name(w27) -> ("Zone temp ref"=w18:variant)
  n473 = call "Close all.vi"("error in (no error)"=w5, "Cameras"=w15) -> ("error out"=w1:errorcluster)  [unwired: 9 in]
  n474 = disable-structure shown="Disabled" {
    frame Disabled {
      (unwired) string[] ["Cookbook Stopped"] ("[user-defined descriptions]")
      w1110 = T26 2 items=["no dialog", "OK message", "continue or stop message", "OK message + warnings", "continue/stop + warnings"] ("type of dialog (OK msg:1)")
      n475 = call <vilib>:"General Error Handler.vi"("[user-defined codes]"=i32[] [5000], "type of dialog (OK msg:1)"=w1110) -> ("[user-defined descriptions]"=w1112:string[])  [unwired: 8 in, 5 out]
      n476 = One Button Dialog(message="Please Enter \nAn Observer\nAnd A Comment") -> ()  [unwired: 1 in, 1 out]
    }
    frame Enabled {
    }
  }
  n477 = Variant To Data(type=refnum<k24> refnum ("ILabVIEW In"), Variant=w18) -> (data=w17:refnum<k24>)  [unwired: 1 in, 1 out]
  n478 = Not A Number/Path/Refnum?(number/path/refnum=w17) -> (NaN/Path/Refnum?=w16:bool)
  n479 = disable-structure shown="Disabled" {
    frame Disabled {
      n480 = property on="Camera R Image" class="IntGraph (strict)"() -> (error out=w1113:errorcluster, "YScale.Maximum"=w1115:dbl)  [unwired: 2 in, 1 out]
      n481 = property on="Camera T Image" class="IntGraph (strict)"(error in=w1113) -> ("YScale.Maximum"=w1114:dbl)  [unwired: 1 in, 2 out]
    }
    frame Enabled {
    }
  }
  n482 = case shown="False" w16 {
    tunnel: [w1117 errorcluster {"status"=FALSE, "code"=0, "source"=""} ("error out")] -> w37
    tunnel: w17 -> [w1116 _]
    frame False {
      n483 = call "Std_Bus_Close_System.vi"("ILabVIEW In"=w1116) -> ("error out"=w1117:errorcluster)  [unwired: 1 in, 17 out]
    }
    frame True {
    }
  }
  n484 = Merge Errors(w1, w37) -> (w33:errorcluster)
  n485 = Unbundle By Name(w33) -> ("status"=w34:bool)
  n486 = call "SCMP - Write log v2.vi"("Error to log"=w33, "data"="Program Ended") -> ("error out"=w4:errorcluster, "Last Log Entry"=w2:string)  [unwired: 7 in, 1 out]
  "Main Loop Error" <- w4
  n487 = local write "Latest Actions"(w2) -> ()
  n488 = And(x=FALSE, y=w34) -> (x .and. y?=→"Program":bool)
  n489 = call "Time Delay2"("error in (no error)"=w4) -> ("error out"=w7:errorcluster)  [unwired: 10 in]
  n490 = disable-structure shown="RUN_TIME_ENGINE==True" {
    disable-tunnel: w7 -> [_ _]
    frame condition #0 {
      n491 = Quit LabVIEW() -> ()  [unwired: 1 in]
    }
    frame condition #1 (active) {
    }
  }
  "Instrument" <- w20
